vi "STED Control V10.vi"() -> ()   [LabVIEW 2014]
uses:
  Type Defs/Image Acquisition Parameters.ctl
  Laser Controls.ctl
  Detectors.ctl
  Type Defs/P541.ctl
  Type Defs/M227.ctl
  Type Defs/P612.ctl
  Type Defs/M686.ctl
  Type Defs/P841.ctl
  Type Defs/ASI.ctl
  Type Defs/N664_V2.ctl
  Type Defs/STED Graph Controls.ctl
  Type Defs/Display Controls.ctl
  FPGA-7842R-Reference.ctl
  Manual Controls V2.ctl
  Scan Parameters.ctl
  <vilib>/Utility/miscctls.llb/LVPositionTypeDef.ctl
  Controls/StageStates.ctl
  Focus Lock/Controls/Standard Action for Focus Lock.ctl
  <vilib>/Utility/miscctls.llb/LVRectTypeDef.ctl
  <vilib>/event_ctls.llb/lveventtype.ctl
  <vilib>/Utility/file.llb/Read From Spreadsheet File (DBL).vi
  <vilib>/Utility/file.llb/Write To Spreadsheet File (DBL).vi
panel:
  in  "Follow Cursor":bool
  in  "Laser Controls 2":T1={"Laser On Time (Ticks)"=16, "Laser Delay (Ticks)"=3}
  out "Channel 6":sgl[][](graph)
  out "Channel 5":sgl[][](graph)
  out "Channel 4":sgl[][](graph)
  out "Channel 3":sgl[][](graph)
  out "Channel 2":sgl[][](graph)
  out "Channel 1":sgl[][](graph)
  in  "Display Controls":T2
  in  "Graph Tools":T3={"Zoom Out"=FALSE, "Zoom In"=FALSE, "Reset Zoom"=FALSE, "Pan Tool"=FALSE, "Show Cursor"=FALSE, "Load File"=FALSE, "Fit Tool"=FALSE, "Smooth Tool"=FALSE, "Merge Tool"=FALSE, "Auto Scale"=FALSE, "Apply Color"=FALSE, "Color Map"=enum."Fire"}
  in  "Shutters":T4
  in  "Upper Objective Z - N664":T5={"Up N664"=FALSE, "Down N664"=FALSE, "Step Size (um)"=0.001, "Position (mm)"=0.0, "Home"=FALSE, "Save"=FALSE} {"Step Size (um)" min=0.001}
  in  "Cavity Translation Z - ASI":T6={"Up ASI"=FALSE, "Down ASI"=FALSE, "Step Size (um)"=0.001, "Z (um)"=0.001, "F (um)"=0.001, "Velocity"=0.001} caption="ASI" {"Velocity" min=0.001; "F (um)" min=0.001; "Z (um)" min=-1500.0 max=1500.0; "Step Size (um)" min=0.001}
  in  "Phase Comp Mirror - P841":T7={"Position (µm)"=0.0, "Step Size (µm)"=1.0, "Up P841"=FALSE, "Down P841"=FALSE}
  in  "Sample Stage XY - M686":T8={"Home Button"=FALSE, "Up Button"=FALSE, "Left Button"=FALSE, "Down Button"=FALSE, "Right Button"=FALSE, "X"=0.0, "Y"=0.0, "Step Size (um)"=1.0} {"Y" format="%#_8g"; "X" format="%#_8g"}
  in  "Bottom Objective XY - P612":T9
  in  "Abort AllStage":bool
  in  "Stages":T10={"M227"=TRUE, "N664"=TRUE, "P612"=TRUE, "M686"=TRUE, "P841"=TRUE, "ASI"=FALSE}
  in  "Sample Z Coarse - M227":T11
  in  "Tab Control":T12(tab)
  in  "SLM":bool
  in  "DM":bool
  in  "Timing":bool
  in  "Camera":bool
  in  "Focus Lock":bool
  in  "Sample Z - P541":T13={"Step Up"=FALSE, "Step Down"=FALSE, "Z Position"=0.0, "Step Size (um)"=1.0, "Home"=FALSE, "Save"=FALSE}
  in  "Detectors":T14={"PMT"=TRUE, "Far Red (685/40 nm)"=FALSE, "Orange (624/40 nm)"=FALSE, "Green (525/50 nm)"=FALSE, "Sum All"=FALSE}
  in  "Laser Controls":T15 {"STED Power (V)" scale=0.0..10.0}
  in  "Save File Path":path=path "C:/isoSTED_Data/Temp/Test_0000.dbl"
  in  "Capture":bool
  in  "Image Acquisition Parameters":T16={"Scan Type"=enum."Beam Scanning", "Scan Mode"=enum."XY", "Fast Axis Frequency (Hz)"=15780.0, "Image Format"=256, "Line Accumulations"=100, "Frames Per Capture"=1, "Frames Accumulations"=1, "Image Dimension (um)"=[15.0, 15.0], "Number of Z Steps"=1, "Z Steps Size (um)"=1.0, "Pixel Size (nm)"=[58.59375, 58.59375]} {"Z Steps Size (um)" min=0.0; "Number of Z Steps" min=1; "Frames Accumulations" min=1; "Frames Per Capture" min=1; "Line Accumulations" min=1; "Image Format" items=["64 x 64"=64, "128 x 128"=128, "256 x 256"=256, "512 x 512"=512, "1024 x 1024"=1024, "2048 x 2048"=2048]}
  in  "Live":bool
  in  "Exit":bool
  # "XY"
  # "Z"
  # "Length"
  # "Height"
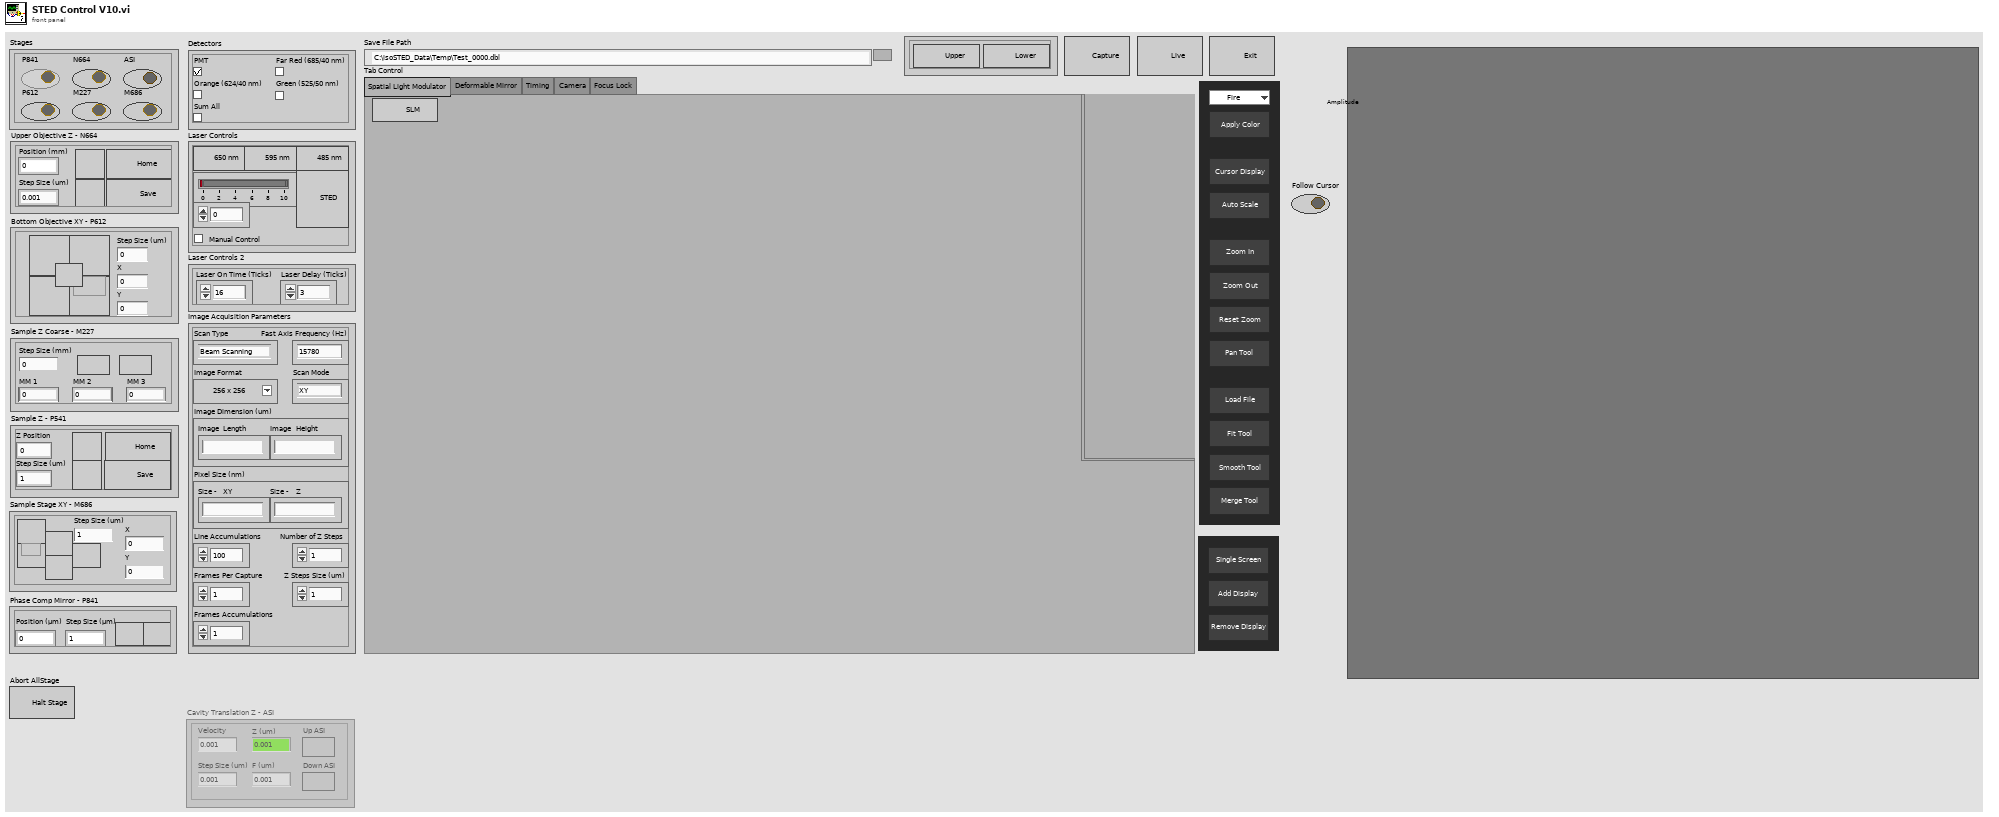
[diagram p1: front panel]
types:
  T1 = cluster{"Laser On Time (Ticks)":i8, "Laser Delay (Ticks)":i8}
  T2 = typedef "Display Controls.ctl" = cluster{"Remove Display":bool, "Add Display":bool, "Single Screen":bool}
  T3 = typedef "STED Graph Controls.ctl" = cluster{"Zoom Out":bool, "Zoom In":bool, "Reset Zoom":bool, "Pan Tool":bool, "Show Cursor":bool, "Load File":bool, "Fit Tool":bool, "Smooth Tool":bool, "Merge Tool":bool, "Auto Scale":bool, "Apply Color":bool, "Color Map":enum16{"System", "Fire", "Gray", "Red", "Green", "Blue", "Cyan", "Magenta", "Yellow", "Red-White", "Green-White", "Blue-White", "Glow"}}
  T4 = cluster{"Upper Shutter":bool, "Lower Shutter":bool}
  T5 = typedef "N664_V2.ctl" = cluster{"Up N664":bool, "Down N664":bool, "Step Size (um)":dbl, "Position (mm)":dbl, "Home":bool, "Save":bool}
  T6 = typedef "ASI.ctl" = cluster{"Up ASI":bool, "Down ASI":bool, "Step Size (um)":dbl, "Z (um)":dbl, "F (um)":dbl, "Velocity":dbl}
  T7 = typedef "P841.ctl" = cluster{"Position (µm)":dbl, "Step Size (µm)":dbl, "Up P841":bool, "Down P841":bool}
  T8 = typedef "M686.ctl" = cluster{"Home Button":bool, "Up Button":bool, "Left Button":bool, "Down Button":bool, "Right Button":bool, "X":dbl, "Y":dbl, "Step Size (um)":dbl}
  T9 = typedef "P612.ctl" = cluster{"Home Button":bool, "Up Button":bool, "Left Button":bool, "Down Button":bool, "Right Button":bool, "Step Size (um)":dbl, "X":dbl, "Y":dbl}
  T10 = cluster{"M227":bool, "N664":bool, "P612":bool, "M686":bool, "P841":bool, "ASI":bool}
  T11 = typedef "M227.ctl" = cluster{"Up M227":bool, "Down M227":bool, "Step Size (mm)":dbl, "MM 1":dbl, "MM 2":dbl, "MM 3":dbl}
  T12 = enum32{"Spatial Light Modulator", "Deformable Mirror", "Timing", "Camera", "Focus Lock"}
  T13 = typedef "P541.ctl" = cluster{"Step Up":bool, "Step Down":bool, "Z Position":dbl, "Step Size (um)":dbl, "Home":bool, "Save":bool}
  T14 = typedef "Detectors.ctl" = cluster{"PMT":bool, "Far Red (685/40 nm)":bool, "Orange (624/40 nm)":bool, "Green (525/50 nm)":bool, "Sum All":bool}
  T15 = typedef "Laser Controls.ctl" = cluster{"STED Power (V)":dbl, "STED":bool, "650 nm":bool, "590 nm":bool, "485 nm":bool, "Manual Control":bool}
  T16 = typedef "Image Acquisition Parameters.ctl" = cluster{"Scan Type":enum16{"Sample Scanning", "Beam Scanning"}, "Scan Mode":enum16{"XY", "XZ", "YZ", "XYZ"}, "Fast Axis Frequency (Hz)":dbl, "Image Format":u16, "Line Accumulations":u16, "Frames Per Capture":u16, "Frames Accumulations":u16, "Image Dimension (um)":dbl[], "Number of Z Steps":u8, "Z Steps Size (um)":dbl, "Pixel Size (nm)":dbl[]}
  T17 = typedef "Scan Parameters.ctl" = cluster{"Fast_Ax_Amp_V":dbl, "Fast_Ax_Off_V":dbl, "Slow_Ax_Amp_V":dbl, "Slow_Ax_Off_V ":dbl, "Slow_Ax_Max_V_VperS":dbl, "Slow_Ax1_Del25ns":i32, "Slow_Ax2_Del25ns":i32, "Stage_X_Off_V":dbl, "Stage_Y_Off_V":dbl, "Stage_Z_Off_V":dbl, "Galvo1_Off_V":dbl, "Galvo2_Off_V":dbl, "Last_Scan_Mode":enum16{"XY", "XZ", "YZ", "XYZ"}, "Current_Scan_Mode":enum16{"XY", "XZ", "YZ", "XYZ"}, "Fly_Back_Lines":u16, "Linear_Ramp_End":u32, "Z_Step_I16":i16, "Z_Start_I16":i16, "Laser_States _U32":u32, "590_Voltage_I16":i16, "775_AOM_Volt_I16":i16, "Blanking OFF":bool, "Unused_Axis_I16":i16}
  T18 = typedef "Manual Controls V2.ctl" = cluster{"Galvo 1 Position (I16)":i16, "Galvo 2 Position (I16)":i16, "X Axis Voltage (I16)":i16, "Y Axis Voltage (I16)":i16, "Z Axis Voltage (I16)":i16, "Res Mirror Amp (I16)":i16, "Res Mirror Mute":bool, "Upper Shutter":bool, "Lower Shutter":bool}
  T19 = typedef "FPGA-7842R-Reference.ctl" = enum16{"Stage Control", "Laser Control", "Unused Axis I16", "Exit", "Set Res Mirror", "Set Galvo", "Current Frame for Capture", "Default", "Close FPGA", "Stop Waveforms", "Start Waveforms", "Shutter Control", "Initialize"}
  T20 = enum8{"Enabled", "Disabled", "Disabled and Grayed Out"}
  T21 = typedef "StageStates.ctl" = enum16{"POSITION", "MVR", "MOVE", "HALT", "ONTARGET", "ERROR", "EXIT", "HOME", "ZEROPOS", "NANOPOS", "QUIT", "ANALOG"}
  T22 = typedef "Standard Action for Focus Lock.ctl" = enum16{"Read", "Write"}
  T23 = typedef "LVRectTypeDef.ctl" = cluster{"Left":i16, "Top":i16, "Right":i16, "Bottom":i16}
  T24 = enum32{"Invalid", "Standard", "Closed", "Hidden", "Minimized", "Maximized"}
  T25 = typedef "lveventtype.ctl" = enum32{"Null", "Timeout", "Annotation Menu Selection", "Annotation Menu Selection?", "App Instance Close", "App Instance Close?", "Autoscale Range Change", "Bookmark Info Change", "Cell Edit", "Cell Edit?", "Cursor Grab", "Cursor Grab?", "Cursor Menu Selection", "Cursor Menu Selection?", "Cursor Move", "Cursor Release", "Data Change", "Direction Change", "Display State Change", "Drag Ended", "Drag Enter", "Drag Leave", "Drag Over", "Drag Source Update", "Drag Starting", "Drag Starting?", "Drop", "Exec State Change", "Key Down", "Key Down?", "Key Repeat", "Key Repeat?", "Key Up", "Listbox Double Click", "Menu Activation?", "Menu Selection (App)", "Menu Selection? (App)", "Menu Selection (User)", "Mouse Down", "Mouse Down?", "Mouse Enter", "Mouse Leave", "Mouse Move", "Mouse Up", "Mouse Wheel", "NI Security User Change (App)", "Pane Size", "Panel Close", "Panel Close?", "Panel Resize", "Plot Attribute Change", "Scale Range Change", "Shortcut Menu Activation?", "Shortcut Menu Selection (App)", "Shortcut Menu Selection? (App)", "Shortcut Menu Selection (User)", "Tree Double Click", "Tree Drag", "Tree Drag?", "Tree Drop", "Tree Drop?", "Tree Item Close", "Tree Item Close?", "Tree Item Open", "Tree Item Open?", "User Event", "Value Change"}
  T26 = typedef "LVPositionTypeDef.ctl" = cluster{"Left":i32, "Top":i32}
  T27 = cluster{"Upper Shutter":bool, "Upper Shutter":bool}
  T28 = cluster{bool, bool, dbl, "Numeric":dbl, "Numeric":dbl, "Numeric":dbl}
  T29 = cluster{"Down_N664":bool, "Down_N664":bool, "Step Size (um)":dbl, "Numeric":dbl, bool, bool}
  T30 = cluster{bool, bool, bool, bool, bool, dbl, "Numeric":dbl, "Numeric":dbl}
  T31 = cluster{bool, bool, bool, bool, bool, "Numeric":dbl, "Numeric":dbl, dbl}
  T32 = cluster{"Scan Type":bool, "Scan Mode":bool, "Fast Axis Frequency (Hz)":bool, "Image Format":bool, "Line Accumulations":bool, "Frames Per Capture":bool, "Frames Accumulations":bool, "Image Dimension (um)":bool[], "Number of Z Steps":bool, "Z Steps Size (um)":bool, "Pixel Size (nm)":bool[]}
  T33 = cluster{"EXIT":bool, "Lock Current":bool, "Correct":bool, "Drift":bool, "Move":bool}
  T34 = typedef "LVAllMonitorsDisplayTypeDef.ctl" = cluster{"Bounds":cluster{"Left":i16, "Top":i16, "Right":i16, "Bottom":i16}, "Depth":i16}[]
  T35 = cluster{"Bounds":cluster{"Left":i16, "Top":i16, "Right":i16, "Bottom":i16}, "Depth":i16}
  T36 = enum16{"System", "Fire", "Gray", "Red", "Green", "Blue", "Cyan", "Magenta", "Yellow", "Red-White", "Green-White", "Blue-White", "Glow"}
  T37 = typedef "LVPointDoubleTypeDef.ctl" = cluster{"Cursor X":dbl, "Cursor Y":dbl}
  T38 = typedef "LVRangeTypeDef.ctl" = cluster{"Minimum":dbl, "Maximum":dbl, "Increment":dbl, "Minor Increment":dbl, "Start":dbl}
  T39 = typedef "IMAQ Image.ctl" = refnum<image>
  T40 = typedef "Waveform Data.ctl" = cluster{"Waveform Scan Parameters":cluster{"Scanning Mode":u8, "Fast Axis WF Length (Elements)":i32, "Fast Axis Sample Period (Ticks)":u32, "Slow Axis 1 WF Length (Elements)":i32, "Slow Axis 1 Sample Period (Ticks)":u32, "Slow Axis 1 Delay (25 ns) Steps":i32, "Slow Axis 2 WFLength (Elements)":i32, "Slow Axis 2 Sample Period (Ticks)":u32, "Slow Axis 2 Delay (25 ns) Steps":i32}, "Fast Axis Waveform":dbl[], "Slow Axis 1 Waveform":dbl[], "Slow Axis 2 Waveform":dbl[]}
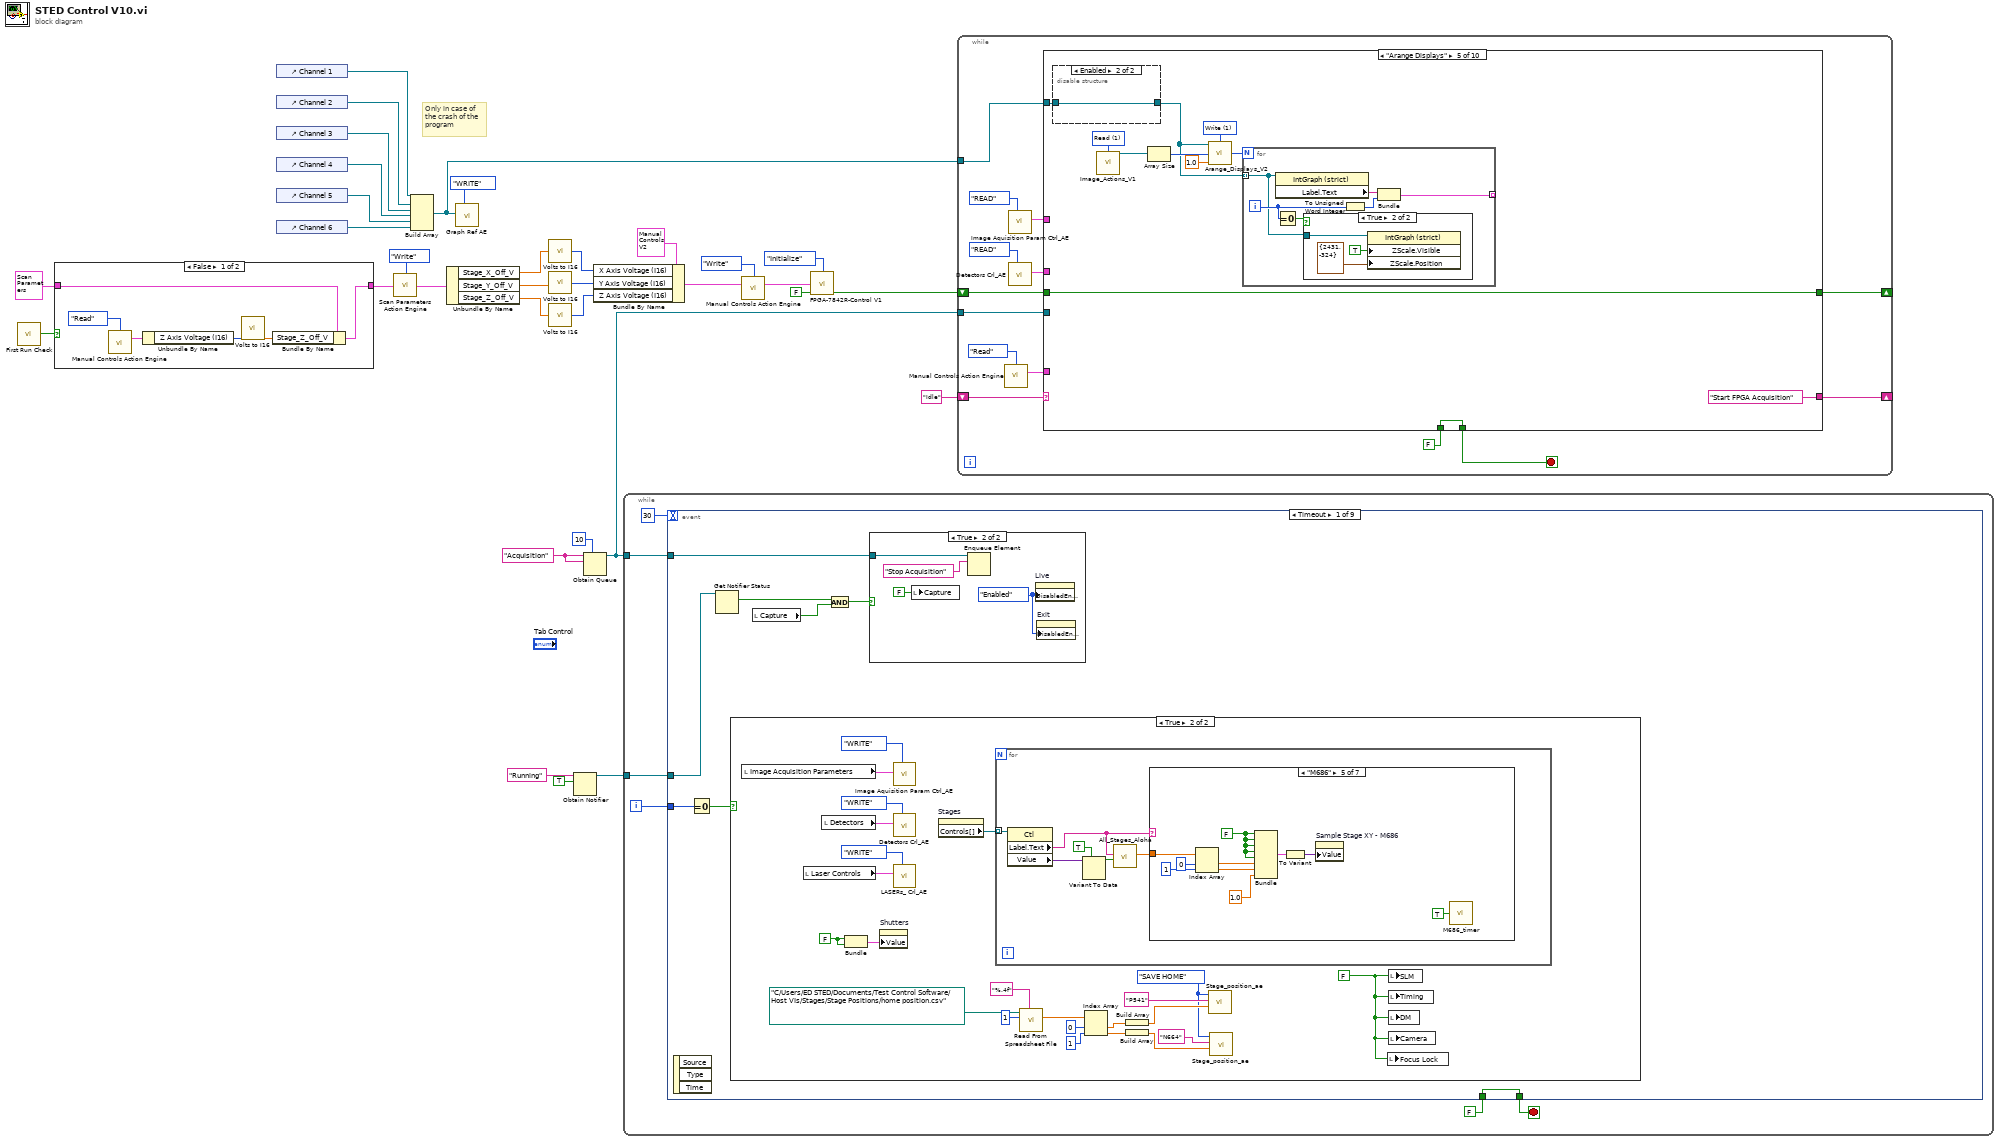
[diagram p0: block diagram]
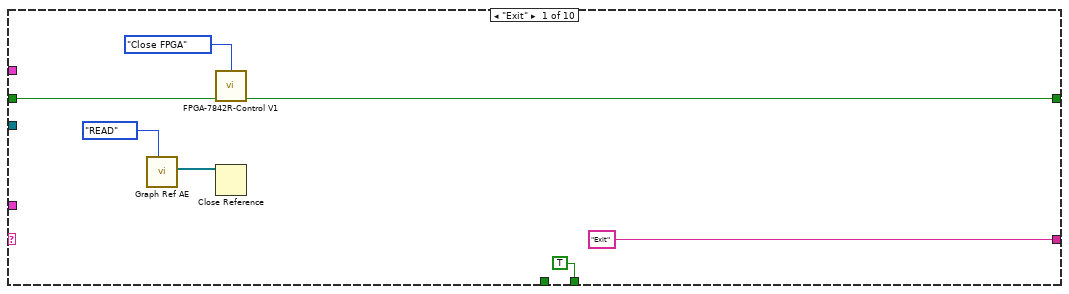
[diagram p3: hidden frame]
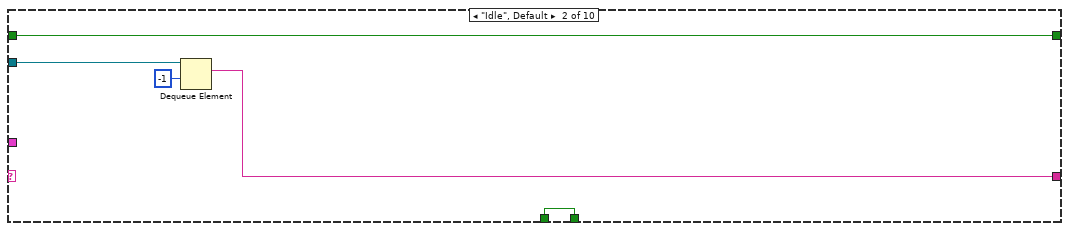
[diagram p4: hidden frame]
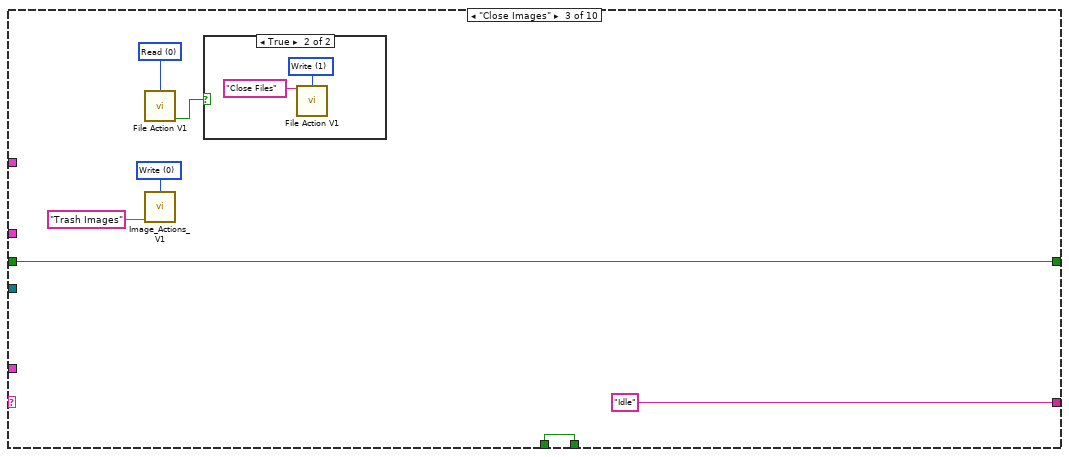
[diagram p5: hidden frame]
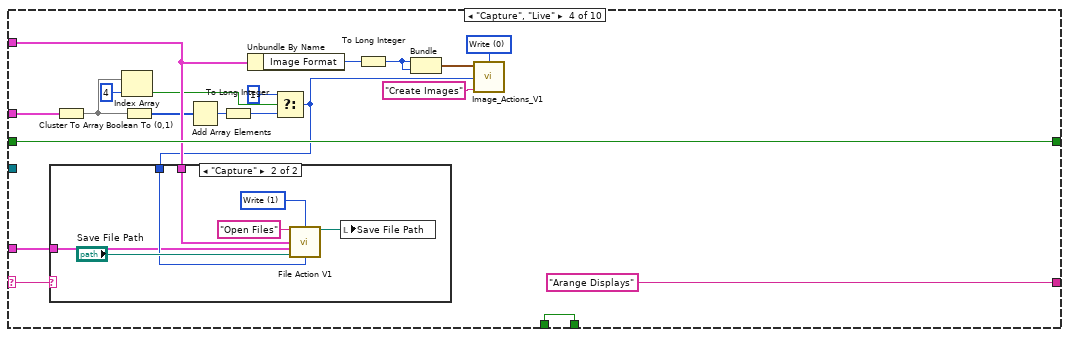
[diagram p7: hidden frame]
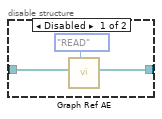
[diagram p9: hidden frame]
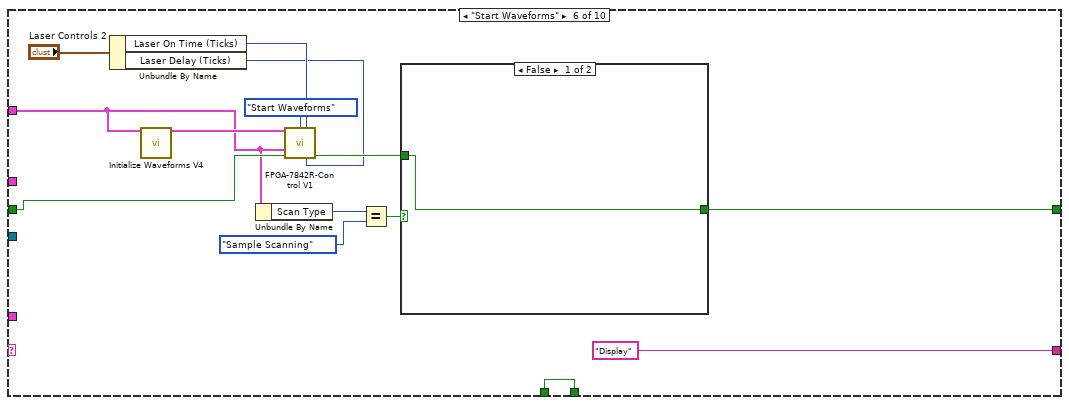
[diagram p11: hidden frame]
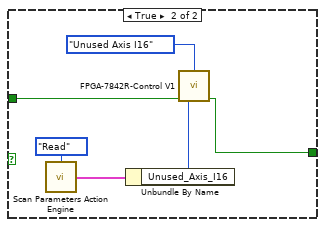
[diagram p12: hidden frame]
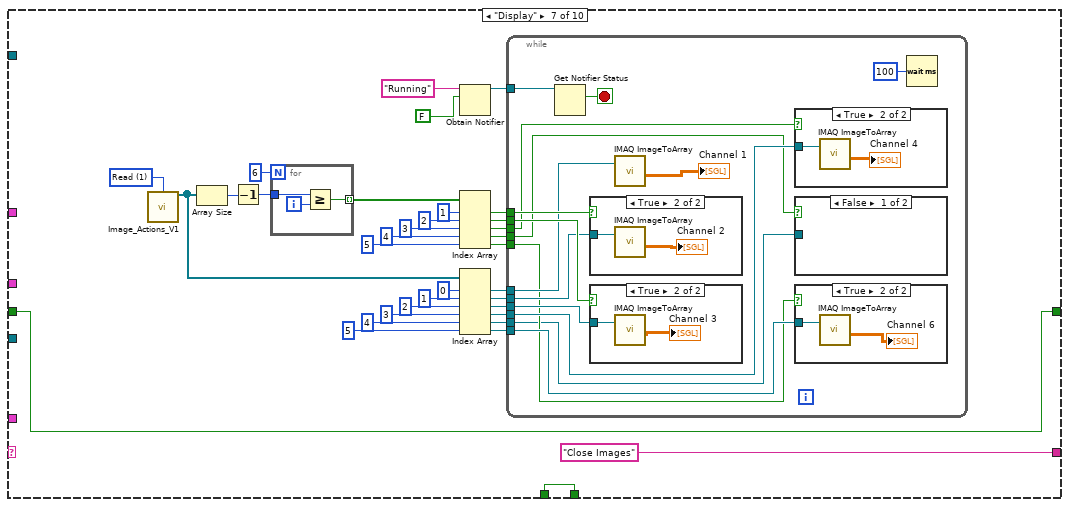
[diagram p13: hidden frame]
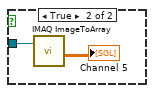
[diagram p15: hidden frame]
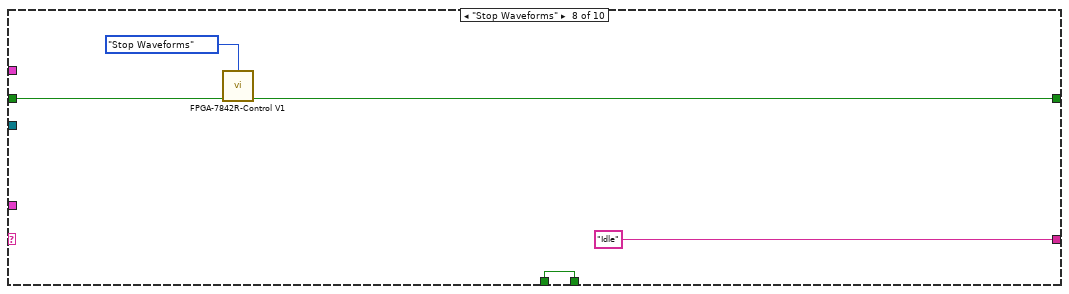
[diagram p19: hidden frame]
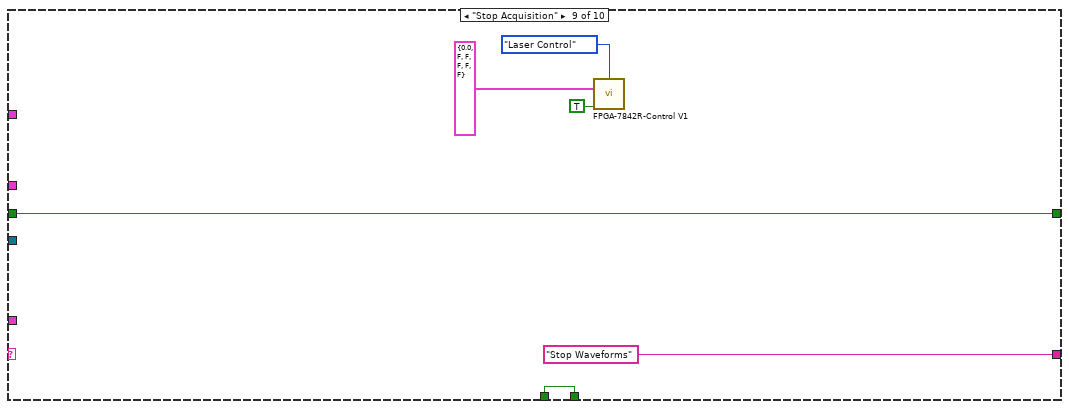
[diagram p20: hidden frame]
diagram:
  w16 = "Acquisition" ("name (unnamed)")
  # "Only in case of \nthe crash of the\nprogram"
  n1 = call "First Run Check.vi"() -> ("First Run?"=w10:bool)  [unwired: 15 in]
  n2 = case shown="False" w10 {
    tunnel: T17 {"Fast_Ax_Amp_V"=0.0, "Fast_Ax_Off_V"=0.0, "Slow_Ax_Amp_V"=0.0, "Slow_Ax_Off_V "=0.0, "Slow_Ax_Max_V_VperS"=0.0, "Slow_Ax1_Del25ns"=0, "Slow_Ax2_Del25ns"=0, "Stage_X_Off_V"=5.0, "Stage_Y_Off_V"=5.0, "Stage_Z_Off_V"=5.0, "Galvo1_Off_V"=0.0, "Galvo2_Off_V"=0.0, "Last_Scan_Mode"=enum."XY", "Current_Scan_Mode"=enum."XY", "Fly_Back_Lines"=0, "Linear_Ramp_End"=0, "Z_Step_I16"=0, "Z_Start_I16"=0, "Laser_States _U32"=0, "590_Voltage_I16"=0, "775_AOM_Volt_I16"=0, "Blanking OFF"=FALSE, "Unused_Axis_I16"=16384} ("Scan Parameters IN") -> [w39 w40]
    tunnel: [w34 w40] -> w8
    frame False {
      n3 = call "Manual Controls Action Engine.vi"("Action"=enum16{"Read", "Write"}."Read") -> ("Manual Controls Out"=w37:T18)  [unwired: 14 in]
      n4 = Unbundle By Name(w37) -> ("Z Axis Voltage (I16)"=w38:i16)
      n5 = call "Volts to I16.vi"("Volatge (I16)"=w38) -> ("Voltage (V)"=w35:dbl)  [unwired: 13 in, 1 out]
      n6 = Bundle By Name(cluster=w39, "Stage_Z_Off_V"=w35) -> (w34:T17)
    }
    frame True {
    }
  }
  n7 = control-ref of="Channel 1"() -> (w5:refnum<vi>)
  n8 = control-ref of="Channel 2"() -> (w6:refnum<vi>)
  n9 = control-ref of="Channel 3"() -> (w7:refnum<vi>)
  n10 = control-ref of="Channel 4"() -> (w2:refnum<vi>)
  n11 = control-ref of="Channel 5"() -> (w4:refnum<vi>)
  n12 = control-ref of="Channel 6"() -> (w3:refnum<vi>)
  n13 = call "Scan Parameters Action Engine.vi"("Action"=enum16{"Read", "Write"}."Write", "Scan Parameters IN"=w8) -> ("Scan Parameters OUT"=w26:T17)  [unwired: 13 in]
  n14 = Build Array(w5, w6, w7, w2, w4, w3) -> (w1:refnum<vi>[])
  n15 = Unbundle By Name(w26) -> ("Stage_X_Off_V"=w22:dbl, "Stage_Y_Off_V"=w21:dbl, "Stage_Z_Off_V"=w20:dbl)
  n16 = call "Graph Ref AE.vi"("Action"=enum16{"READ", "WRITE"}."WRITE", "Graph Ref In"=w1) -> ()  [unwired: 9 in, 1 out]
  n17 = call "Volts to I16.vi"("Voltage (V)"=w22) -> ("I16"=w23:i16)  [unwired: 13 in, 1 out]
  n18 = call "Volts to I16.vi"("Voltage (V)"=w21) -> ("I16"=w24:i16)  [unwired: 13 in, 1 out]
  n19 = call "Volts to I16.vi"("Voltage (V)"=w20) -> ("I16"=w25:i16)  [unwired: 13 in, 1 out]
  n20 = Obtain Notifier(name (unnamed)="Running", notification data type=TRUE) -> (notifier out=w12:refnum<notifier>)  [unwired: 2 in, 2 out]
  n21 = Obtain Queue(max queue size (-1, unlimited)=10, name (unnamed)=w16, element data type=w16) -> (queue out=w18:refnum<queue>)  [unwired: 2 in, 2 out]
  n22 = Bundle By Name(cluster=T18 {"Galvo 1 Position (I16)"=-280, "Galvo 2 Position (I16)"=0, "X Axis Voltage (I16)"=16384, "Y Axis Voltage (I16)"=16384, "Z Axis Voltage (I16)"=16384, "Res Mirror Amp (I16)"=0, "Res Mirror Mute"=FALSE, "Upper Shutter"=FALSE, "Lower Shutter"=FALSE} ("Manual Controls"), "X Axis Voltage (I16)"=w23, "Y Axis Voltage (I16)"=w24, "Z Axis Voltage (I16)"=w25) -> (w27:T18)
  n23 = while {
    tunnel: w18 -> [w44]
    tunnel: w12 -> [w41]
    i -> [w42]
    stop <- w46 stop-if-true
    n24 = event shown="[0] Timeout" {
      selector: _ -> [_ _ _ _ _ _ _ _ _]
      dyn-events: _ -> [_ _ _ _ _ _ _ _ _]
      timeout: 30 -> [_ _ _ _ _ _ _ _ _]
      tunnel: [w54 w189 w202 w367 _ w714 w795 w999 w1052] -> w46
      tunnel: FALSE -> [w54 w189 w202 w367 _ w714 w795 w999 _]
      tunnel: w44 -> [w51 w188 _ _ _ _ _ _ w1051]
      tunnel: w42 -> [w49 _ _ _ _ _ _ _ _]
      tunnel: w41 -> [w47 w181 _ _ _ _ _ _ w1045]
      event Timeout {
        n25 = event-data() -> ()  [unwired: 1 in, 3 out]
        n26 = Equal To 0?(x=w49) -> (x = 0?=w48:bool)
        n27 = Get Notifier Status(notifier=w47) -> (current notification=w53:bool)  [unwired: 1 in, 4 out]
        n28 = case shown="True" w48 {
          frame False {
            w61 = enum16{"WRITE", "READ", "HOME", "SAVE HOME"}."READ" ("Enum")
            n29 = call "Image Aquisition Param Ctrl_AE.vi"("Action"=enum16{"READ", "WRITE"}."READ") -> ("Image Acquisition Parameters Out"=w89:T16)  [unwired: 10 in]
            n30 = call "Detectors Crl_AE.vi"("Action"=enum16{"READ", "WRITE"}."READ") -> ("Detectors Parameters Out"=w90:T14)  [unwired: 10 in]
            n31 = call "LASERs_ Crl_AE.vi"("Action"=enum16{"READ", "WRITE"}."READ") -> ("Detectors Parameters Out"=w91:T15)  [unwired: 10 in]
            n32 = local write "Image Acquisition Parameters"(w89) -> ()
            n33 = local write "Detectors"(w90) -> ()
            n34 = local write "Laser Controls"(w91) -> ()
            n35 = call "Stage_position_ae.vi"("StageID"="M686", "Enum"=w61) -> ("Position Out"=w59:dbl[])  [unwired: 8 in, 1 out]
            n36 = call "Stage_position_ae.vi"("StageID"="M227", "Enum"=w61) -> ("Position Out"=w67:dbl[])  [unwired: 8 in, 1 out]
            n37 = call "Stage_position_ae.vi"("StageID"="P612", "Enum"=w61) -> ("Position Out"=w84:dbl[])  [unwired: 8 in, 1 out]
            n38 = call "Stage_position_ae.vi"("StageID"="P841", "Enum"=w61) -> ("Position Out"=w77:dbl[])  [unwired: 8 in, 1 out]
            n39 = call "Stage_position_ae.vi"("StageID"="N664", "Enum"=w61) -> ("Position Out"=w71:dbl[])  [unwired: 8 in, 1 out]
            n40 = Index Array(array=w71, index=0) -> (element=w70:dbl)
            n41 = Index Array(array=w77, index=0) -> (element=w74:dbl)
            n42 = Index Array(array=w84, index #1=0 ("index"), index #2=1 ("index"), index #3=2 ("index")) -> (element #1=w83:dbl, element #2=w80:dbl, element #3=w78:dbl)
            n43 = Index Array(array=w59, index #1=0 ("index"), index #2=1 ("index")) -> (element #1=w56:dbl, element #2=w55:dbl)
            n44 = Index Array(array=w67, index #1=0 ("index"), index #2=1 ("index"), index #3=2 ("index")) -> (element #1=w64:dbl, element #2=w63:dbl, element #3=w62:dbl)
            n45 = property on="Position (µm)" class="DigNum (strict)"("Value"=w74) -> ()  [unwired: 2 in, 2 out]
            n46 = property on="Position (mm)" class="DigNum (strict)"("Value"=w70) -> ()  [unwired: 2 in, 2 out]
            n47 = property on="X" class="DigNum (strict)"("Value"=w83) -> ()  [unwired: 2 in, 2 out]
            n48 = property on="Y" class="DigNum (strict)"("Value"=w80) -> ()  [unwired: 2 in, 2 out]
            n49 = property on="X" class="DigNum (strict)"("Value"=w56) -> ()  [unwired: 2 in, 2 out]
            n50 = property on="MM 1" class="DigNum (strict)"("Value"=w64) -> ()  [unwired: 2 in, 2 out]
            n51 = property on="MM 2" class="DigNum (strict)"("Value"=w63) -> ()  [unwired: 2 in, 2 out]
            n52 = property on="Z Position" class="DigNum (strict)"("Value"=w78) -> ()  [unwired: 2 in, 2 out]
            n53 = property on="Y" class="DigNum (strict)"("Value"=w55) -> ()  [unwired: 2 in, 2 out]
            n54 = property on="MM 3" class="DigNum (strict)"("Value"=w62) -> ()  [unwired: 2 in, 2 out]
          }
          frame True {
            w92 = FALSE ("SLM")
            w94 = enum16{"WRITE", "READ", "HOME", "SAVE HOME"}."SAVE HOME" ("Enum")
            w106 = FALSE ("Upper Shutter")
            n55 = local read "Image Acquisition Parameters"() -> (w113:T16)
            n56 = local read "Laser Controls"() -> (w111:T15)
            n57 = local read "Detectors"() -> (w110:T14)
            n58 = Bundle("Upper Shutter"=w106, "Upper Shutter"=w106) -> (w107:T27)  [unwired: 1 in]
            n59 = property on="Shutters" class="Clust (strict)"("Value"=w107) -> ()  [unwired: 2 in, 2 out]
            n60 = call "Image Aquisition Param Ctrl_AE.vi"("Action"=enum16{"READ", "WRITE"}."WRITE", "Image Acquisition Parameters In"=w113) -> ()  [unwired: 9 in, 1 out]
            n61 = call "Detectors Crl_AE.vi"("Action"=enum16{"READ", "WRITE"}."WRITE", "Detectors Parameters In"=w110) -> ()  [unwired: 9 in, 1 out]
            n62 = call "LASERs_ Crl_AE.vi"("Action"=enum16{"READ", "WRITE"}."WRITE", "Detectors Parameters In"=w111) -> ()  [unwired: 9 in, 1 out]
            n63 = property on="Stages" class="Clust (strict)"() -> ("Controls[]"=w108:refnum<vi>[])  [unwired: 2 in, 2 out]
            n64 = for {
              tunnel: w108 -> [w118] mode=indexing
              n65 = property class="Ctl"(reference=w118) -> ("Label.Text"=w116:string, "Value"=w120:variant)  [unwired: 1 in, 2 out]
              n66 = Variant To Data(type=TRUE, Variant=w120) -> (data=w117:bool)  [unwired: 1 in, 1 out]
              n67 = call "All_Stages_Aloha.vi"("Aloha"=w117, "Stage ID"=w116) -> ("Position Out"=w115:dbl[])  [unwired: 9 in]
              n68 = case shown="\"M686\"" w116 {
                tunnel: w115 -> [_ w127 w135 w142 w151 w162 w172]
                frame "0", Default {
                }
                frame "M227" {
                  w131 = FALSE
                  n69 = Index Array(array=w127, index #1=0 ("index"), index #2=1 ("index"), index #3=2 ("index")) -> (element #1=w123:dbl, element #2=w122:dbl, element #3=w121:dbl)
                  n70 = Bundle(w131, w131, 0.0, "Numeric"=w123, "Numeric"=w122, "Numeric"=w121) -> (w129:T28)  [unwired: 1 in]
                  n71 = To Variant(anything=w129) -> (Variant=w128:variant)
                  n72 = property on="Sample Z Coarse - M227" class="Clust"("Value"=w128) -> ()  [unwired: 2 in, 2 out]
                }
                frame "N664" {
                  w132 = FALSE
                  w138 = FALSE ("Down_N664")
                  n73 = Index Array(array=w135, index=0) -> (element=w136:dbl)
                  n74 = Bundle("Down_N664"=w138, "Down_N664"=w138, "Step Size (um)"=1.0, "Numeric"=w136, w132, w132) -> (w134:T29)  [unwired: 1 in]
                  n75 = To Variant(anything=w134) -> (Variant=w133:variant)
                  n76 = property on="Upper Objective Z - N664" class="Clust"("Value"=w133) -> ()  [unwired: 2 in, 2 out]
                }
                frame "P612" {
                  w150 = FALSE
                  n77 = Index Array(array=w142, index #1=0, index #2=1, index #3=2 ("index")) -> (element #1=w147:dbl, element #2=w145:dbl, element #3=w140:dbl)
                  n78 = Bundle(w150, w150, w150, w150, w150, 1.0, "Numeric"=w147, "Numeric"=w145) -> (w146:T30)  [unwired: 1 in]
                  n79 = To Variant(anything=w146) -> (Variant=w141:variant)
                  n80 = property on="Bottom Objective XY - P612" class="Clust"("Value"=w141) -> ()  [unwired: 2 in, 2 out]
                  n81 = property on="Z Position" class="DigNum (strict)"("Value"=w140) -> ()  [unwired: 2 in, 2 out]
                }
                frame "M686" {
                  w160 = FALSE
                  n82 = Index Array(array=w151, index #1=0, index #2=1) -> (element #1=w155:dbl, element #2=w154:dbl)
                  n83 = Bundle(w160, w160, w160, w160, w160, "Numeric"=w155, "Numeric"=w154, 1.0) -> (w158:T31)  [unwired: 1 in]
                  n84 = To Variant(anything=w158) -> (Variant=w156:variant)
                  n85 = property on="Sample Stage XY - M686" class="Clust"("Value"=w156) -> ()  [unwired: 2 in, 2 out]
                  n86 = call "M686_timer.vi"("Reset"=TRUE) -> ()  [unwired: 1 out]
                }
                frame "P841" {
                  n87 = Index Array(array=w162, index=0) -> (element=w161:dbl)
                  n88 = property on="Position (µm)" class="DigNum (strict)"("Value"=w161) -> ()  [unwired: 2 in, 2 out]
                }
                frame "ASI" {
                  w168 = FALSE
                  n89 = Add Array Elements(numeric array=w172) -> (sum=w174:dbl)
                  n90 = Index Array(array=w172, index #1=0 ("index"), index #2=1 ("index")) -> (element #1=w167:dbl, element #2=w166:dbl)
                  n91 = Divide(x=w174, y=2000.0) -> ()  [unwired: 1 out]
                  n92 = Bundle By Name(cluster=T6 {"Up ASI"=FALSE, "Down ASI"=FALSE, "Step Size (um)"=0.001, "Z (um)"=0.001, "F (um)"=0.001, "Velocity"=0.001} ("Cavity Translation Z - ASI"), "Up ASI"=w168, "Down ASI"=w168, "Step Size (um)"=1.0, "Z (um)"=w167, "F (um)"=w166, "Velocity"=0.1) -> (w164:T6)
                  n93 = To Variant(anything=w164) -> (Variant=w165:variant)
                  n94 = property on="Cavity Translation Z - ASI" class="Clust"("Value"=w165) -> ()  [unwired: 2 in, 2 out]
                }
              }
            }
            n95 = call-poly <vilib>:"Read From Spreadsheet File.vi"("format (%.3f)"="%.4f", "number of rows (all:-1)"=1, "file path (dialog if empty)"=path "C:/Users/ED STED/Documents/Test Control Software/Host VIs/Stages/Stage Positions/home position.csv") -> ("first row"=w103:dbl[])  [unwired: 4 in, 4 out]
            n96 = Index Array(array=w103, index #1=0 ("index"), index #2=1 ("index")) -> (element #1=w99:dbl, element #2=w100:dbl)
            n97 = Build Array(w99) -> (w98:dbl[])
            n98 = Build Array(w100) -> (w96:dbl[])
            n99 = call "Stage_position_ae.vi"("Position In"=w98, "StageID"="P541", "Enum"=w94) -> ()  [unwired: 7 in, 2 out]
            n100 = call "Stage_position_ae.vi"("Position In"=w96, "StageID"="N664", "Enum"=w94) -> ()  [unwired: 7 in, 2 out]
            n101 = local write "Focus Lock"(w92) -> ()
            n102 = local write "SLM"(w92) -> ()
            n103 = local write "Timing"(w92) -> ()
            n104 = local write "DM"(w92) -> ()
            n105 = local write "Camera"(w92) -> ()
          }
        }
        n106 = local read "Capture"() -> (w52:bool)
        n107 = And(x=w53, y=w52) -> (x .and. y?=w50:bool)
        n108 = case shown="True" w50 {
          tunnel: w51 -> [_ w179]
          frame False {
          }
          frame True {
            w177 = T20."Enabled" ("Disabled")
            n109 = local write "Capture"(FALSE ("Capture")) -> ()
            n110 = Enqueue Element(queue=w179, element="Stop Acquisition" ("f")) -> ()  [unwired: 2 in, 3 out]
            n111 = property on="Live" class="Bool (strict)"("DisabledEnum"=w177) -> ()  [unwired: 2 in, 2 out]
            n112 = property on="Exit" class="Bool"("DisabledEnum"=w177) -> ()  [unwired: 2 in, 2 out]
          }
        }
      }
      event "Live", "Capture": Value Change {
        n113 = event-data() -> ("CtlRef"=w187:refnum<vi>, "NewVal"=w182:bool)  [unwired: 1 in]
        n114 = Not(x=w182) -> (.not. x?=w185:bool)
        n115 = property class="Bool (strict)"(reference=w187) -> ("Label.Text"=w183:string)  [unwired: 1 in, 2 out]
        n116 = Send Notification(notification=w185, notifier=w181) -> ()  [unwired: 1 in, 2 out]
        n117 = case shown="\"Capture\"" w183 {
          tunnel: w182 -> [_ w191 w194]
          frame "False", Default {
          }
          frame "Live" {
            n118 = case shown="True" w191 {
              tunnel: [T20."Enabled" ("Disabled") T20."Disabled and Grayed Out" ("Disabled")] -> w190
              frame False {
              }
              frame True {
              }
            }
            n119 = property on="Capture" class="Bool (strict)"("DisabledEnum"=w190) -> ()  [unwired: 2 in, 2 out]
            n120 = property on="Exit" class="Bool"("DisabledEnum"=w190) -> ()  [unwired: 2 in, 2 out]
          }
          frame "Capture" {
            n121 = case shown="True" w194 {
              tunnel: [T20."Enabled" ("Disabled") T20."Disabled and Grayed Out" ("Disabled")] -> w195
              frame False {
              }
              frame True {
              }
            }
            n122 = property on="Live" class="Bool (strict)"("DisabledEnum"=w195) -> ()  [unwired: 2 in, 2 out]
            n123 = property on="Exit" class="Bool"("DisabledEnum"=w195) -> ()  [unwired: 2 in, 2 out]
          }
        }
        n124 = Select(t=w183, s=w182, f="Stop Acquisition") -> (s? t:f=w184:string)
        n125 = Enqueue Element(queue=w188, element=w184) -> ()  [unwired: 2 in, 3 out]
      }
      event "Shutters": Value Change {
        n126 = event-data() -> ("CtlRef"=w201:refnum<vi>, "NewVal"=w200:variant, "OldVal"=w199:variant)  [unwired: 1 in]
        n127 = property class="Clust"(reference=w201) -> ("Label.Text"=w198:string)  [unwired: 1 in, 2 out]
        n128 = case shown="\"Image Acquisition Parameters\"" w198 {
          tunnel: w200 -> [_ w217 _ _ _]
          tunnel: w199 -> [_ w215 _ _ _]
          frame Default {
          }
          frame "Image Acquisition Parameters" {
            n129 = Variant To Data(type="Image Acquisition Parameters", Variant=w217) -> (data=w214:T16)  [unwired: 1 in, 1 out]
            n130 = Variant To Data(type=w214, Variant=w215) -> (data=w213:T16)  [unwired: 1 in, 1 out]
            n131 = Not Equal?(x=w214, y=w213) -> (x != y?=w238:T32)
            n132 = Unbundle By Name(w238) -> ("Image Dimension (um)"=w223:bool[], "Image Format"=w221:bool, "Pixel Size (nm)"=w222:bool[], "Scan Mode"=w204:bool)
            n133 = Or Array Elements(Boolean array=w223) -> (logical OR=w227:bool)
            n134 = Or Array Elements(Boolean array=w222) -> (logical OR=w226:bool)
            n135 = Build Array(w227, w221, w226) -> (w225:bool[])
            n136 = Boolean Array To Number(Boolean array=w225) -> (number=w224:u32)
            n137 = case shown="1, 2" w224 {
              tunnel: w223 -> [_ w288 _]
              tunnel: w214 -> [w276 w281 w296]
              tunnel: [w276 w279 w294] -> w220
              tunnel: w222 -> [_ _ w293]
              tunnel: [w275 w278 w292] -> w219
              tunnel: [w274 w277 w291] -> w206
              frame 0, Default {
                n138 = Unbundle By Name(w276) -> ("Image Dimension (um)"=w275:dbl[], "Scan Mode"=w274:enum16{"XY", "XZ", "YZ", "XYZ"})
              }
              frame 1, 2 {
                # "Image Dimension or Format Change"
                n139 = Unbundle By Name(w281) -> ("Image Dimension (um)"=w287:dbl[], "Image Format"=w285:u16, "Scan Mode"=w277:enum16{"XY", "XZ", "YZ", "XYZ"})
                n140 = for {
                  tunnel: w288 -> [w290] mode=indexing
                  tunnel: w287 -> [w289] mode=indexing
                  tunnel: [w289] -> w286
                  stop <- w290 stop-if-true
                }
                n141 = To Double Precision Float(number=w285) -> (double precision float=w284:dbl)
                n142 = Build Array(w286, w286) -> (w278:dbl[])
                n143 = Divide(x=w278, y=w284) -> (x/y=w283:dbl[])
                n144 = Multiply(x=w283, y=1000.0) -> (x*y=w280:dbl[])
                n145 = Bundle By Name(cluster=w281, "Image Dimension (um)"=w278, "Pixel Size (nm)"=w280) -> (w279:T16)
              }
              frame 4 {
                # "Pixel Size Change"
                n146 = Unbundle By Name(w296) -> ("Pixel Size (nm)"=w302:dbl[], "Image Format"=w300:u16, "Scan Mode"=w291:enum16{"XY", "XZ", "YZ", "XYZ"})
                n147 = for {
                  tunnel: w293 -> [w304] mode=indexing
                  tunnel: w302 -> [w303] mode=indexing
                  tunnel: [w303] -> w301
                  stop <- w304 stop-if-true
                }
                n148 = Build Array(w301, w301) -> (w295:dbl[])
                n149 = To Double Precision Float(number=w300) -> (double precision float=w299:dbl)
                n150 = Multiply(x=w295, y=w299) -> (x*y=w298:dbl[])
                n151 = Multiply(x=w298, y=0.001) -> (x*y=w292:dbl[])
                n152 = Bundle By Name(cluster=w296, "Pixel Size (nm)"=w295, "Image Dimension (um)"=w292) -> (w294:T16)
              }
            }
            n153 = And(x=w204, y="Follow Cursor") -> (x .and. y?=w203:bool)
            n154 = case shown="True" w203 {
              tunnel: w206 -> [_ w248]
              frame False {
              }
              frame True {
                n155 = Not Equal?(x=w248, y=enum16{"XY", "XZ", "YZ", "XYZ"}."XZ") -> (x != y?=w246:bool)
                n156 = case shown="True" w246 {
                  frame False {
                    n157 = call "Y Slice.vi"() -> ("Y position"=w256:dbl)  [unwired: 1 in]
                    n158 = Build Array(0.0 ("element"), w256) -> (w254:dbl[])
                    n159 = call "AllStage_Limits_Array.vi"("Step(um)/Position(units)"=w254, "Axis"=bool[] [TRUE, TRUE, TRUE], "Stage ID"="M686", "MOVE/MVR"=enum16{"MOVE", "MVR"}."MVR") -> ("Positions"=w250:dbl[], "Boolean Array"=w251:bool[], "Stage ID"=w252:string)  [unwired: 4 in, 1 out]
                    n160 = call "AE_AllStages_Action V2.vi"("Velocity"=0.0, "Positions"=w250, "Axis"=w251, "Stage ID"=w252, "Action"=StageStates."MVR") -> ()  [unwired: 4 in, 3 out]
                  }
                  frame True {
                    n161 = call "Z Slice.vi"() -> ("Y position"=w270:dbl)  [unwired: 1 in]
                    n162 = call "Manual Controls Action Engine.vi"("Action"=enum16{"Read", "Write"}."Read") -> ("Manual Controls Out"=w265:T18)  [unwired: 14 in]
                    n163 = Multiply(x=w270, y=327.68) -> (x*y=w272:dbl)
                    n164 = Round To Nearest(number=w272) -> (nearest integer value=w271:dbl)
                    n165 = Unbundle By Name(w265) -> ("Z Axis Voltage (I16)"=w268:i16)
                    n166 = To Word Integer(number=w271) -> (16bit integer=w267:i16)
                    n167 = Add(x=w268, y=w267) -> (x+y=w266:i16)
                    n168 = Bundle By Name(cluster=w265, "Z Axis Voltage (I16)"=w266) -> (w264:T18)
                    n169 = call "Manual Controls Action Engine.vi"("Action"=enum16{"Read", "Write"}."Write", "Manual Controls In"=w264) -> ("Manual Controls Out"=w262:T18)  [unwired: 13 in]
                    n170 = call "FPGA-7842R-Control V1.vi"("Action"=FPGA-7842R-Reference."Stage Control", "Manual Controls"=w262, "Initialize"=TRUE) -> ()  [unwired: 11 in, 2 out]
                  }
                }
              }
            }
            n171 = Index Array(array=w219, index=0) -> (element=w243:dbl)
            n172 = Not Equal?(x=enum16{"XY", "XZ", "YZ", "XYZ"}."YZ" ("y"), y=w206) -> (x != y?=w228:bool)
            n173 = call "Res Mirror um to Volts.vi"("Image Size (um)"=w243) -> ("Voltage (V)"=w207:dbl)
            n174 = Select(t=15780.0, s=w228, f=200.0) -> (s? t:f=w231:dbl)
            n175 = In Range and Coerce(upper limit=5.0, x=w207, lower limit=0.0) -> (coerced(x)=w209:dbl)  [unwired: 1 out]
            n176 = call "Scan Parameters Action Engine.vi"("Action"=enum16{"Read", "Write"}."Read") -> ("Scan Parameters OUT"=w210:T17)  [unwired: 14 in]
            n177 = Bundle By Name(cluster=w210, "Fast_Ax_Amp_V"=w209) -> (w208:T17)
            n178 = Bundle By Name(cluster=w220, "Fast Axis Frequency (Hz)"=w231) -> (w230:T16)
            n179 = call "Volts to I16.vi"("Voltage (V)"=w209) -> ("I16"=w242:i16)  [unwired: 13 in, 1 out]
            n180 = call "Scan Parameters Action Engine.vi"("Action"=enum16{"Read", "Write"}."Write", "Scan Parameters IN"=w208) -> ()  [unwired: 13 in, 1 out]
            n181 = call "Manual Controls Action Engine.vi"("Action"=enum16{"Read", "Write"}."Read") -> ("Manual Controls Out"=w236:T18)  [unwired: 14 in]
            n182 = Bundle By Name(cluster=w236, "Res Mirror Amp (I16)"=w242, "Res Mirror Mute"=w228) -> (w234:T18)
            n183 = call "Image Aquisition Param Ctrl_AE.vi"("Action"=enum16{"READ", "WRITE"}."WRITE", "Image Acquisition Parameters In"=w230) -> ()  [unwired: 9 in, 1 out]
            n184 = call "FPGA-7842R-Control V1.vi"("Action"=FPGA-7842R-Reference."Set Res Mirror", "Manual Controls"=w234, "Initialize"=TRUE) -> ()  [unwired: 11 in, 2 out]
            n185 = call "Manual Controls Action Engine.vi"("Action"=enum16{"Read", "Write"}."Write", "Manual Controls In"=w234) -> ()  [unwired: 13 in, 1 out]
          }
          frame "Detectors" {
            n186 = call "Detectors Crl_AE.vi"("Action"=enum16{"READ", "WRITE"}."WRITE", "Detectors Parameters In"="Detectors") -> ()  [unwired: 9 in, 1 out]
          }
          frame "Laser Controls" {
            w319 = FALSE ("element")
            n187 = Unbundle By Name("Laser Controls") -> ("STED"=w325:bool, "650 nm"=w322:bool, "590 nm"=w323:bool, "485 nm"=w324:bool, "STED Power (V)"=w316:dbl, "Manual Control"=w308:bool)
            n188 = local read "Live"() -> (w311:bool)
            n189 = call "LASERs_ Crl_AE.vi"("Action"=enum16{"READ", "WRITE"}."WRITE", "Detectors Parameters In"="Laser Controls") -> ()  [unwired: 9 in, 1 out]
            n190 = Or(x=w311, y=w308) -> (x .or. y?=w310:bool)
            n191 = In Range and Coerce(upper limit=10.0, x=w316, lower limit=0.0) -> (coerced(x)=w313:dbl)  [unwired: 1 out]
            n192 = Build Array(w325, w322, w323, w324, w319, w319, w319, w319) -> (w321:bool[])
            n193 = case shown="True" w310 {
              tunnel: "Laser Controls" -> [_ w339]
              frame False {
              }
              frame True {
                n194 = call "FPGA-7842R-Control V1.vi"("Action"=FPGA-7842R-Reference."Laser Control", "Laser Controls"=w339, "Initialize"=TRUE) -> ()  [unwired: 11 in, 2 out]
              }
            }
            n195 = Boolean Array To Number(Boolean array=w321) -> (number=w320:u32)
            n196 = To Unsigned Byte Integer(number=w320) -> (unsigned 8bit integer=w318:u8)
            n197 = call "U8_To_U32.vi"("U8 IN"=w318) -> ("U32 OUT"=w317:u32)  [unwired: 13 in, 1 out]
            n198 = call "Volts to I16.vi"("Voltage (V)"=w313) -> ("I16"=w312:i16)  [unwired: 13 in, 1 out]
            n199 = case shown="False" w308 {
              tunnel: "Laser Controls" -> [w337 _]
              frame False {
                n200 = Unbundle By Name(w337) -> ("650 nm"=w334:bool, "590 nm"=w333:bool, "485 nm"=w332:bool)
                n201 = call "Detectors Crl_AE.vi"("Action"=enum16{"READ", "WRITE"}."READ") -> ("Detectors Parameters Out"=w335:T14)  [unwired: 10 in]
                n202 = Bundle By Name(cluster=w335, "Far Red (685/40 nm)"=w334, "Orange (624/40 nm)"=w333, "Green (525/50 nm)"=w332) -> (w331:T14)
                n203 = call "Detectors Crl_AE.vi"("Action"=enum16{"READ", "WRITE"}."WRITE", "Detectors Parameters In"=w331) -> ()  [unwired: 9 in, 1 out]
              }
              frame True {
              }
            }
            n204 = call "Scan Parameters Action Engine.vi"("Action"=enum16{"Read", "Write"}."Read") -> ("Scan Parameters OUT"=w328:T17)  [unwired: 14 in]
            n205 = Bundle By Name(cluster=w328, "Laser_States _U32"=w317, "775_AOM_Volt_I16"=w312) -> (w326:T17)
            n206 = call "Scan Parameters Action Engine.vi"("Action"=enum16{"Read", "Write"}."Write", "Scan Parameters IN"=w326) -> ()  [unwired: 13 in, 1 out]
          }
          frame "Shutters" {
            n207 = Unbundle By Name("Shutters") -> ("Upper Shutter"=w351:bool, "Lower Shutter"=w350:bool)
            n208 = Not(x=w351) -> (.not. x?=w342:bool)
            n209 = Not(x=w350) -> (.not. x?=w341:bool)
            n210 = call "Manual Controls Action Engine.vi"("Action"=enum16{"Read", "Write"}."Read") -> ("Manual Controls Out"=w346:T18)  [unwired: 14 in]
            n211 = Bundle By Name(cluster=w346, "Upper Shutter"=w342, "Lower Shutter"=w341) -> (w343:T18)
            n212 = call "Manual Controls Action Engine.vi"("Action"=enum16{"Read", "Write"}."Write", "Manual Controls In"=w343) -> ()  [unwired: 13 in, 1 out]
            n213 = call "FPGA-7842R-Control V1.vi"("Action"=FPGA-7842R-Reference."Shutter Control", "Manual Controls"=w343, "Initialize"=TRUE) -> ()  [unwired: 11 in, 2 out]
          }
        }
      }
      event Value Change {
        # "For P541 - Sample Z - Converting from Step in µm to I16 is as follows. We have (Step µw)*(10 V / 100 µm)*(32768 I16 / 10 V) = (Step µm)*(32768 I16 / 100 µm) = (Step µm)*(327.68 I16/µm)"
        n214 = event-data() -> ("CtlRef"=w365:refnum<vi>, "OldVal"=w363:variant, "NewVal"=w364:variant)  [unwired: 1 in]
        n215 = local write "Abort AllStage"(FALSE ("Abort AllStage")) -> ()
        n216 = property class="Clust"(reference=w365) -> ("Label.Text"=w362:string)  [unwired: 1 in, 2 out]
        n217 = case shown="\"Sample Z - P541\"" w362 {
          tunnel: w364 -> [_ w388 w429 w456 w519 w560 w589 w628]
          tunnel: w363 -> [_ w387 w428 w455 w520 w561 w590 w629]
          tunnel: ["" "N664" "ASI" "P612" "P612" "P841" "M227" "M686"] -> w361
          tunnel: [dbl[] [0.0] w379 w421 w444 dbl[] [0.0] w549 w582 w618] -> w360
          tunnel: [bool[] [FALSE] w377 w415 w445 bool[] [FALSE] bool[] [TRUE] w583 w617] -> w359
          tunnel: [enum16{"MOVE", "MVR"}."MVR" ("MOVE/MVR") w376 w418 w447 enum16{"MOVE", "MVR"}."MVR" ("MOVE/MVR") w552 w575 w620] -> w358
          tunnel: [0.0 ("Step Size (um)") 0.5 ("Step Size (um)") w420 0.0 ("Velocity") 0.0 ("Velocity") 10000.0 ("Velocity") 0.0 ("Velocity") 0.0 ("Velocity")] -> w354
          tunnel: [StageStates."MVR" ("Action") w374 w419 w448 StageStates."POSITION" ("Action") w553 w579 w621] -> w352
          frame Default {
          }
          frame "Upper Objective Z - N664" {
            n218 = call "N664_Ctrl_Index.vi"("OldVal"=w387, "NewVal"=w388) -> ("Control Ref OUT"=w386:refnum<vi>, "N664 Out"=w384:T5)  [unwired: 12 in]
            n219 = property class="Ctl"(reference=w386) -> ("Label.Text"=w385:string)  [unwired: 1 in, 2 out]
            n220 = Unbundle By Name(w384) -> ("Step Size (um)"=w383:dbl, "Position (mm)"=w382:dbl)
            n221 = case shown="\"Home\"" w385 {
              tunnel: w383 -> [_ w393 w396 _ _ _]
              tunnel: [0.0 ("Step Size (um)") w392 w396 w401 w403 w408] -> w380
              tunnel: w382 -> [_ _ _ w401 w403 _]
              tunnel: [enum16{"MOVE", "MVR"}."MVR" ("MOVE/MVR") enum16{"MOVE", "MVR"}."MVR" ("MOVE/MVR") enum16{"MOVE", "MVR"}."MVR" ("MOVE/MVR") enum16{"MOVE", "MVR"}."MOVE" ("MOVE/MVR") enum16{"MOVE", "MVR"}."MOVE" ("MOVE/MVR") enum16{"MOVE", "MVR"}."MOVE" ("MOVE/MVR")] -> w376
              tunnel: [StageStates."MVR" ("Action") StageStates."MVR" ("Action") StageStates."MVR" ("Action") StageStates."MOVE" ("Action") StageStates."MOVE" ("Action") StageStates."MOVE" ("Action")] -> w374
              frame Default {
              }
              frame "Up N664" {
                n222 = Negate(x=w393) -> (-x=w392:dbl)
              }
              frame "Down N664" {
              }
              frame "Position (mm)" {
              }
              frame "Save" {
                n223 = Build Array(w403) -> (w402:dbl[])
                n224 = call "Stage_position_ae.vi"("Position In"=w402, "StageID"="N664", "Enum"=enum16{"WRITE", "READ", "HOME", "SAVE HOME"}."SAVE HOME") -> ()  [unwired: 7 in, 2 out]
              }
              frame "Home" {
                n225 = call "Stage_position_ae.vi"("StageID"="N664", "Enum"=enum16{"WRITE", "READ", "HOME", "SAVE HOME"}."HOME") -> ("Position Out"=w410:dbl[])  [unwired: 8 in, 1 out]
                n226 = Index Array(array=w410, index=0) -> (element=w408:dbl)
              }
            }
            n227 = Build Array(w380) -> (w379:dbl[])
            n228 = Build Array(TRUE) -> (w377:bool[])
          }
          frame "Cavity Translation Z - ASI" {
            n229 = call "ASI_Ctrl_Index.vi"("NewVal"=w429, "OldVal"=w428) -> ("ASI out"=w425:T6, "Control Ref OUT"=w427:refnum<vi>)  [unwired: 8 in]
            n230 = property class="Ctl"(reference=w427) -> ("Label.Text"=w426:string)  [unwired: 1 in, 2 out]
            n231 = Unbundle By Name(w425) -> ("Step Size (um)"=w424:dbl, "Z (um)"=w423:dbl, "Velocity"=w420:dbl)
            n232 = case shown="\"Z (um)\"" w426 {
              tunnel: w424 -> [_ w435 w438 _]
              tunnel: w423 -> [_ _ _ w442]
              tunnel: [0.0 ("Z (um)") w435 w439 w442] -> w422
              tunnel: [StageStates."MVR" ("Action") StageStates."MVR" ("Action") StageStates."MVR" ("Action") StageStates."MOVE" ("Action")] -> w419
              tunnel: [enum16{"MOVE", "MVR"}."MVR" ("MOVE/MVR") enum16{"MOVE", "MVR"}."MVR" ("MOVE/MVR") enum16{"MOVE", "MVR"}."MVR" ("MOVE/MVR") enum16{"MOVE", "MVR"}."MOVE" ("MOVE/MVR")] -> w418
              frame Default {
              }
              frame "Up ASI" {
              }
              frame "Down ASI" {
                n233 = Negate(x=w438) -> (-x=w439:dbl)
              }
              frame "Z (um)" {
              }
            }
            n234 = Build Array(w422) -> (w421:dbl[])
            n235 = Build Array(TRUE) -> (w415:bool[])
          }
          frame "Bottom Objective XY - P612" {
            n236 = call "P612_Ctrl_Index.vi"("OldVal"=w455, "NewVal"=w456) -> ("Control out"=w454:refnum<vi>, "P612 out"=w452:T9)  [unwired: 12 in]
            n237 = property class="Ctl"(reference=w454) -> ("Label.Text"=w453:string)  [unwired: 1 in, 2 out]
            n238 = Unbundle By Name(w452) -> ("Step Size (um)"=w451:dbl, "X"=w450:dbl, "Y"=w449:dbl)
            n239 = case shown="\"Up Button\"" w453 {
              tunnel: w451 -> [_ _ w467 w474 w478 w485 _]
              tunnel: w450 -> [_ _ _ _ _ _ w492]
              tunnel: w449 -> [_ _ _ _ _ _ w491]
              tunnel: [StageStates."MVR" ("Action") StageStates."HOME" ("Action") StageStates."MVR" ("Action") StageStates."MVR" ("Action") StageStates."MVR" ("Action") StageStates."MVR" ("Action") StageStates."MOVE" ("Action")] -> w448
              tunnel: [enum16{"MOVE", "MVR"}."MVR" ("MOVE/MVR") enum16{"MOVE", "MVR"}."MVR" ("MOVE/MVR") enum16{"MOVE", "MVR"}."MVR" ("MOVE/MVR") enum16{"MOVE", "MVR"}."MVR" ("MOVE/MVR") enum16{"MOVE", "MVR"}."MVR" ("MOVE/MVR") enum16{"MOVE", "MVR"}."MVR" ("MOVE/MVR") enum16{"MOVE", "MVR"}."MOVE" ("MOVE/MVR")] -> w447
              tunnel: [bool[] [FALSE] bool[] [TRUE, TRUE] bool[] [TRUE, FALSE] bool[] [TRUE, FALSE] bool[] [FALSE, TRUE] bool[] [FALSE, TRUE] bool[] [TRUE, TRUE]] -> w445
              tunnel: [dbl[] [0.0] dbl[] [0.0, 0.0] w466 w473 w480 w487 w493] -> w444
              frame Default {
              }
              frame "Home Button" {
              }
              frame "Up Button" {
                n240 = Build Array(w467, 0.0 ("element")) -> (w466:dbl[])
              }
              frame "Down Button" {
                n241 = Negate(x=w474) -> (-x=w471:dbl)
                n242 = Build Array(w471, 0.0 ("element")) -> (w473:dbl[])
              }
              frame "Left Button" {
                n243 = Build Array(0.0 ("element"), w478) -> (w480:dbl[])
              }
              frame "Right Button" {
                n244 = Negate(x=w485) -> (-x=w484:dbl)
                n245 = Build Array(0.0 ("element"), w484) -> (w487:dbl[])
              }
              frame "X", "Y" {
                n246 = Build Array(w492, w491) -> (w493:dbl[])
              }
            }
          }
          frame "Sample Z - P541" {
            w498 = 327.68 ("y")
            n247 = call "P541_Ctrl_Index.vi"("OldVal"=w520, "NewVal"=w519) -> ("Control out"=w518:refnum<vi>, "P541 Out"=w517:T13)  [unwired: 12 in]
            n248 = Unbundle By Name(w517) -> ("Z Position"=w497:dbl, "Step Size (um)"=w516:dbl)
            n249 = property class="Ctl"(reference=w518) -> ("Label.Text"=w515:string)  [unwired: 1 in, 2 out]
            n250 = call "Manual Controls Action Engine.vi"("Action"=enum16{"Read", "Write"}."Read") -> ("Manual Controls Out"=w506:T18)  [unwired: 14 in]
            n251 = Unbundle By Name(w506) -> ("Z Axis Voltage (I16)"=w509:i16)
            n252 = Multiply(x=w497, y=w498) -> (x*y=w512:dbl)
            n253 = Multiply(x=w516, y=w498) -> (x*y=w514:dbl)
            n254 = Round To Nearest(number=w512) -> (nearest integer value=w501:dbl)
            n255 = Round To Nearest(number=w514) -> (nearest integer value=w500:dbl)
            n256 = To Word Integer(number=w501) -> (16bit integer=w511:i16)
            n257 = To Word Integer(number=w500) -> (16bit integer=w513:i16)
            n258 = case shown="\"Step Up\"" w515 {
              tunnel: w513 -> [_ w527 w531 _ _ _]
              tunnel: w511 -> [_ _ _ w533 _ _]
              tunnel: w509 -> [w526 w529 w532 _ w538 _]
              tunnel: [w526 w528 w530 w533 w538 w544] -> w505
              tunnel: w498 -> [_ _ _ _ _ w543]
              tunnel: w497 -> [_ _ _ _ w537 _]
              frame Default {
              }
              frame "Step Down" {
                n259 = Subtract(x=w529, y=w527) -> (x-y=w528:i16)
              }
              frame "Step Up" {
                n260 = Add(x=w532, y=w531) -> (x+y=w530:i16)
              }
              frame "Z Position" {
              }
              frame "Save" {
                n261 = Build Array(w537) -> (w536:dbl[])
                n262 = call "Stage_position_ae.vi"("Position In"=w536, "StageID"="P541", "Enum"=enum16{"WRITE", "READ", "HOME", "SAVE HOME"}."SAVE HOME") -> ()  [unwired: 7 in, 2 out]
              }
              frame "Home" {
                n263 = call "Stage_position_ae.vi"("StageID"="P541", "Enum"=enum16{"WRITE", "READ", "HOME", "SAVE HOME"}."HOME") -> ("Position Out"=w541:dbl[])  [unwired: 8 in, 1 out]
                n264 = Index Array(array=w541, index=0) -> (element=w539:dbl)
                n265 = Multiply(x=w539, y=w543) -> (x*y=w545:dbl)
                n266 = Round To Nearest(number=w545) -> (nearest integer value=w546:dbl)
                n267 = To Word Integer(number=w546) -> (16bit integer=w544:i16)
              }
            }
            n268 = Bundle By Name(cluster=w506, "Z Axis Voltage (I16)"=w505) -> (w508:T18)
            n269 = call "Manual Controls Action Engine.vi"("Action"=enum16{"Read", "Write"}."Write", "Manual Controls In"=w508) -> ("Manual Controls Out"=w502:T18)  [unwired: 13 in]
            n270 = call "FPGA-7842R-Control V1.vi"("Action"=FPGA-7842R-Reference."Stage Control", "Manual Controls"=w502, "Initialize"=TRUE) -> ()  [unwired: 11 in, 2 out]
          }
          frame "Phase Comp Mirror - P841" {
            n271 = call "P841_Ctrl_Index.vi"("OldVal"=w561, "NewVal"=w560) -> ("Control out"=w558:refnum<vi>, "P841 Out"=w556:T7)  [unwired: 12 in]
            n272 = property class="Ctl"(reference=w558) -> ("Label.Text"=w557:string)  [unwired: 1 in, 2 out]
            n273 = Unbundle By Name(w556) -> ("Position (µm)"=w555:dbl, "Step Size (µm)"=w554:dbl)
            n274 = case shown="\"Down P841\"" w557 {
              tunnel: w555 -> [_ _ _ w574]
              tunnel: w554 -> [_ w567 w571 _]
              tunnel: [0.0 ("Position (µm)") w567 w570 w574] -> w550
              tunnel: [StageStates."MVR" ("Action") StageStates."MVR" ("Action") StageStates."MVR" ("Action") StageStates."MOVE" ("Action")] -> w553
              tunnel: [enum16{"MOVE", "MVR"}."MVR" ("MOVE/MVR") enum16{"MOVE", "MVR"}."MVR" ("MOVE/MVR") enum16{"MOVE", "MVR"}."MVR" ("MOVE/MVR") enum16{"MOVE", "MVR"}."MOVE" ("MOVE/MVR")] -> w552
              frame Default {
              }
              frame "Up P841" {
              }
              frame "Down P841" {
                n275 = Negate(x=w571) -> (-x=w570:dbl)
              }
              frame "Position (µm)" {
              }
            }
            n276 = Build Array(w550) -> (w549:dbl[])
          }
          frame "Sample Z Coarse - M227" {
            n277 = call "M227_Ctrl_Index.vi"("OldVal"=w590, "NewVal"=w589) -> ("Control Ref OUT"=w588:refnum<vi>, "M227 Out"=w586:T11)  [unwired: 12 in]
            n278 = property class="Ctl"(reference=w588) -> ("Label.Text"=w587:string)  [unwired: 1 in, 2 out]
            n279 = Unbundle By Name(w586) -> ("Step Size (mm)"=w585:dbl, "MM 1"=w578:dbl, "MM 2"=w577:dbl, "MM 3"=w576:dbl)
            n280 = case shown="\"MM 1\"" w587 {
              tunnel: w585 -> [_ _ _ _ w609 w614]
              tunnel: [bool[] [FALSE, FALSE, FALSE] bool[] [TRUE, TRUE, TRUE] bool[] [TRUE, TRUE, TRUE] bool[] [TRUE, TRUE, TRUE] bool[] [TRUE, TRUE, TRUE] bool[] [TRUE, TRUE, TRUE]] -> w583
              tunnel: [0.0 ("Step Size (mm)") w596 w600 w604 w609 w613] -> w580
              tunnel: [StageStates."POSITION" ("Action") StageStates."MOVE" ("Action") StageStates."MOVE" ("Action") StageStates."MOVE" ("Action") StageStates."MVR" ("Action") StageStates."MVR" ("Action")] -> w579
              tunnel: w578 -> [_ w596 _ _ _ _]
              tunnel: w577 -> [_ _ w600 _ _ _]
              tunnel: w576 -> [_ _ _ w604 _ _]
              tunnel: [enum16{"MOVE", "MVR"}."MVR" ("MOVE/MVR") enum16{"MOVE", "MVR"}."MOVE" ("MOVE/MVR") enum16{"MOVE", "MVR"}."MOVE" ("MOVE/MVR") enum16{"MOVE", "MVR"}."MOVE" ("MOVE/MVR") enum16{"MOVE", "MVR"}."MVR" ("MOVE/MVR") enum16{"MOVE", "MVR"}."MVR" ("MOVE/MVR")] -> w575
              frame Default {
              }
              frame "MM 1" {
              }
              frame "MM 2" {
              }
              frame "MM 3" {
              }
              frame "Up M227" {
              }
              frame "Down M227" {
                n281 = Negate(x=w614) -> (-x=w613:dbl)
              }
            }
            n282 = Build Array(w580, w580, w580) -> (w582:dbl[])
          }
          frame "Sample Stage XY - M686" {
            n283 = call "M686_Ctrl_Index.vi"("NewVal"=w628, "OldVal"=w629) -> ("M686 - out"=w626:T8, "Control out"=w627:refnum<vi>)  [unwired: 8 in]
            n284 = Unbundle By Name(w626) -> ("Step Size (um)"=w625:dbl, "X"=w624:dbl, "Y"=w623:dbl)
            n285 = property class="Ctl"(reference=w627) -> ("Label.Text"=w616:string)  [unwired: 1 in, 2 out]
            n286 = case shown="\"Left Button\"" w616 {
              tunnel: w625 -> [_ _ w641 w646 w654 w659 _]
              tunnel: w624 -> [_ _ _ _ _ _ w666]
              tunnel: w623 -> [_ _ _ _ _ _ w665]
              tunnel: [StageStates."POSITION" ("Action") StageStates."MOVE" ("Action") StageStates."MVR" ("Action") StageStates."MVR" ("Action") StageStates."MVR" ("Action") StageStates."MVR" ("Action") StageStates."MOVE" ("Action")] -> w621
              tunnel: [enum16{"MOVE", "MVR"}."MVR" ("MOVE/MVR") enum16{"MOVE", "MVR"}."MOVE" ("MOVE/MVR") enum16{"MOVE", "MVR"}."MVR" ("MOVE/MVR") enum16{"MOVE", "MVR"}."MVR" ("MOVE/MVR") enum16{"MOVE", "MVR"}."MVR" ("MOVE/MVR") enum16{"MOVE", "MVR"}."MVR" ("MOVE/MVR") enum16{"MOVE", "MVR"}."MOVE" ("MOVE/MVR")] -> w620
              tunnel: [w631 dbl[] [12.5, 12.5] w639 w647 w655 w661 w667] -> w618
              tunnel: [bool[] [FALSE, FALSE] bool[] [TRUE, TRUE] bool[] [TRUE, TRUE] bool[] [TRUE, TRUE] bool[] [TRUE, TRUE] bool[] [TRUE, TRUE] bool[] [TRUE, TRUE]] -> w617
              frame Default {
                w632 = 0.0 ("Step Size (mm)")
                n287 = Build Array(w632, w632) -> (w631:dbl[])
              }
              frame "Home Button" {
              }
              frame "Right Button" {
                n288 = Build Array(w641, 0.0 ("element")) -> (w639:dbl[])
              }
              frame "Left Button" {
                n289 = Negate(x=w646) -> (-x=w645:dbl)
                n290 = Build Array(w645, 0.0 ("element")) -> (w647:dbl[])
              }
              frame "Up Button" {
                n291 = Negate(x=w654) -> (-x=w653:dbl)
                n292 = Build Array(0.0 ("element"), w653) -> (w655:dbl[])
              }
              frame "Down Button" {
                n293 = Build Array(0.0 ("element"), w659) -> (w661:dbl[])
              }
              frame "X", "Y" {
                n294 = Build Array(w666, w665) -> (w667:dbl[])
              }
            }
          }
        }
        n295 = case shown="Default" w362 {
          frame Default {
          }
          frame "Upper Objective Z - N664" {
            n296 = while {
              i -> [w676]
              stop <- w672 stop-if-true
              n297 = call "Stage_position_ae.vi"("StageID"="N664", "Enum"=enum16{"WRITE", "READ", "HOME", "SAVE HOME"}."READ") -> ("Status Out"=w673:bool, "Position Out"=w683:dbl[])  [unwired: 8 in]
              n298 = Greater?(x=w676, y=200) -> (0:w675:bool)
              n299 = And(x=w673, y=w675) -> (x .and. y?=w672:bool)
              n300 = Wait (ms)(milliseconds to wait=u32 1) -> ()  [unwired: 1 out]
              n301 = Index Array(array=w683, index=0) -> (element=w682:dbl)
              n302 = Select(t=u32 16777215, s=w672, f=u32 6618880) -> (s? t:f=w677:u32)
              n303 = property on="Position (mm)" class="DigNum (strict)"("Value"=w682, "NumText.BG Color"=w677) -> ()  [unwired: 2 in, 2 out]
            }
          }
          frame "Cavity Translation Z - ASI" {
            n304 = while {
              shift-right: [w690] -> _
              shift-left: TRUE ("Status Out") -> [w695]
              stop <- w694 stop-if-true
              n305 = call "Stage_position_ae.vi"("StageID"="ASI", "Enum"=enum16{"WRITE", "READ", "HOME", "SAVE HOME"}."READ") -> ("Status Out"=w690:bool, "Position Out"=w698:dbl[])  [unwired: 8 in]
              n306 = Greater?(x=w690, y=w695) -> (0:w694:bool)
              n307 = Wait (ms)(milliseconds to wait=u32 1) -> ()  [unwired: 1 out]
              n308 = Index Array(array=w698, index=0) -> (element=w688:dbl)
              n309 = Divide(x=w688, y=10.0) -> (x/y=w689:dbl)
              n310 = Select(t=u32 16777215, s=w690, f=u32 6618880) -> (s? t:f=w691:u32)
              n311 = property on="Z (um)" class="DigNum (strict)"("Value"=w689, "NumText.BG Color"=w691) -> ()  [unwired: 2 in, 2 out]
            }
          }
        }
        n312 = control-ref of="Abort AllStage"() -> (w353:refnum<vi>)
        n313 = call "AllStage_Limits_Array.vi"("Step(um)/Position(units)"=w360, "Axis"=w359, "Stage ID"=w361, "MOVE/MVR"=w358) -> ("Positions"=w356:dbl[], "Boolean Array"=w355:bool[], "Stage ID"=w357:string)  [unwired: 4 in, 1 out]
        n314 = call "AE_AllStages_Action V2.vi"("Velocity"=w354, "Abort"=w353, "Positions"=w356, "Axis"=w355, "Stage ID"=w357, "Action"=w352) -> ()  [unwired: 3 in, 3 out]
      }
      event "Stages": Value Change {
        n315 = event-data() -> ("NewVal"=w712:T10)  [unwired: 1 in, 2 out]
        n316 = Unbundle By Name(w712) -> ("M686"=w700:bool, "P841"=w710:bool, "ASI"=w708:bool, "N664"=w706:bool, "P612"=w704:bool, "M227"=w702:bool)
        n317 = call "All_Stages_Aloha.vi"("Aloha"=w700, "Stage ID"="M686") -> ()  [unwired: 9 in, 1 out]
        n318 = call "All_Stages_Aloha.vi"("Aloha"=w710, "Stage ID"="P841") -> ()  [unwired: 9 in, 1 out]
        n319 = call "All_Stages_Aloha.vi"("Aloha"=w708, "Stage ID"="ASI") -> ()  [unwired: 9 in, 1 out]
        n320 = call "All_Stages_Aloha.vi"("Aloha"=w706, "Stage ID"="N664") -> ()  [unwired: 9 in, 1 out]
        n321 = call "All_Stages_Aloha.vi"("Aloha"=w704, "Stage ID"="P612") -> ()  [unwired: 9 in, 1 out]
        n322 = call "All_Stages_Aloha.vi"("Aloha"=w702, "Stage ID"="M227") -> ()  [unwired: 9 in, 1 out]
      }
      event "SLM", "Timing", "DM", "Camera", "Focus Lock": Value Change {
        n323 = event-data() -> ("CtlRef"=w716:refnum<vi>, "NewVal"=w713:bool)  [unwired: 1 in, 1 out]
        n324 = property class="Bool (strict)"(reference=w716) -> ("Label.Text"=w715:string)  [unwired: 1 in, 2 out]
        n325 = case shown="\"Focus Lock\"" w715 {
          tunnel: w713 -> [w717 w731 w745 w759 w772]
          frame "SLM", Default {
            n326 = case shown="True" w717 {
              frame False {
                n327 = To Variant(anything=TRUE) -> (Variant=w723:variant)
                n328 = call "SLM AE.vi"("Action"=enum16{"READ", "WRITE"}."READ") -> ("SLM Ref Out"=w724:refnum<vi>)  [unwired: 10 in]
                n329 = invoke class="VI" method="Ctrl Val.Set"(reference=w724, "Control Name"="Exit", "Value"=w723) -> (reference out=w720:refnum<vi>, error out=w719:errorcluster)  [unwired: 2 in, 3 out]
                n330 = invoke on="Hamamatsu LCOS" class="SubPnl" method="Remove VI"(error in=w719) -> (error out=w718:errorcluster)  [unwired: 2 in, 2 out]
                n331 = Close Reference(reference=w720, error in (no error)=w718) -> ()  [unwired: 1 out]
              }
              frame True {
                n332 = Open VI Reference(vi path=path "C:/Users/ED STED/Documents/Test Control Software/Host VIs/SLM_V2/SLM Control.vi") -> (vi reference=w729:refnum<vi>)  [unwired: 5 in, 1 out]
                n333 = invoke class="VI" method="Run VI"(reference=w729, "Wait until done"=FALSE ("Wait Until Done")) -> (reference out=w726:refnum<vi>)  [unwired: 3 in, 4 out]
                n334 = invoke on="Hamamatsu LCOS" class="SubPanel" method="Insert VI"("VI Ref"=w726) -> ()  [unwired: 3 in, 4 out]
                n335 = call "SLM AE.vi"("Action"=enum16{"READ", "WRITE"}."WRITE", "SLM Ref In"=w726) -> ()  [unwired: 9 in, 1 out]
              }
            }
          }
          frame "DM" {
            n336 = case shown="False" w731 {
              frame False {
                n337 = call "DM_Ref_AE.vi"("Action"=enum16{"READ", "WRITE"}."READ") -> ("DM Ref Out"=w738:refnum<vi>)  [unwired: 10 in]
                n338 = To Variant(anything=TRUE) -> (Variant=w737:variant)
                n339 = invoke class="VI" method="Ctrl Val.Set"(reference=w738, "Control Name"="Exit", "Value"=w737) -> (reference out=w734:refnum<vi>, error out=w733:errorcluster)  [unwired: 2 in, 3 out]
                n340 = invoke on="BM Multi" class="SubPnl" method="Remove VI"(error in=w733) -> (error out=w732:errorcluster)  [unwired: 2 in, 2 out]
                n341 = Close Reference(reference=w734, error in (no error)=w732) -> ()  [unwired: 1 out]
              }
              frame True {
                n342 = Open VI Reference(vi path=path "C:/Users/ED STED/Documents/Test Control Software/Host VIs/DM_Dual_V2/Dual_DM_Control_Main_V4.vi") -> (vi reference=w743:refnum<vi>)  [unwired: 5 in, 1 out]
                n343 = invoke class="VI" method="Run VI"(reference=w743, "Wait until done"=FALSE ("Wait Until Done")) -> (reference out=w740:refnum<vi>)  [unwired: 3 in, 4 out]
                n344 = invoke on="BM Multi" class="SubPanel" method="Insert VI"("VI Ref"=w740) -> ()  [unwired: 3 in, 4 out]
                n345 = call "DM_Ref_AE.vi"("Action"=enum16{"READ", "WRITE"}."WRITE", "DM Ref In"=w740) -> ()  [unwired: 9 in, 1 out]
              }
            }
          }
          frame "Timing" {
            n346 = case shown="True" w745 {
              frame False {
                n347 = To Variant(anything=TRUE) -> (Variant=w750:variant)
                n348 = call "GateDelay AE.vi"("Action"=enum16{"READ", "WRITE"}."READ") -> ("Gate Delay Ref Out"=w751:refnum<vi>)  [unwired: 10 in]
                n349 = invoke class="VI" method="Ctrl Val.Set"(reference=w751, "Control Name"="Exit", "Value"=w750) -> (reference out=w746:refnum<vi>, error out=w747:errorcluster)  [unwired: 2 in, 3 out]
                n350 = invoke on="Timing" class="SubPnl" method="Remove VI"(error in=w747) -> (error out=w753:errorcluster)  [unwired: 2 in, 2 out]
                n351 = Close Reference(reference=w746, error in (no error)=w753) -> ()  [unwired: 1 out]
              }
              frame True {
                n352 = Open VI Reference(vi path=path "C:/Users/ED STED/Documents/Test Control Software/Host VIs/Time Delay/GateDelay_Control_V2.vi") -> (vi reference=w756:refnum<vi>)  [unwired: 5 in, 1 out]
                n353 = invoke class="VI" method="Run VI"(reference=w756, "Wait until done"=FALSE ("Wait Until Done")) -> (reference out=w755:refnum<vi>)  [unwired: 3 in, 4 out]
                n354 = invoke on="Timing" class="SubPanel" method="Insert VI"("VI Ref"=w755) -> ()  [unwired: 3 in, 4 out]
                n355 = call "GateDelay AE.vi"("Action"=enum16{"READ", "WRITE"}."WRITE", "Gate Delay Ref In"=w755) -> ()  [unwired: 9 in, 1 out]
              }
            }
          }
          frame "Camera" {
            n356 = case shown="True" w759 {
              frame False {
                n357 = To Variant(anything=TRUE) -> (Variant=w760:variant)
                n358 = call "Camera_Ref_HX.vi"("Action"=enum16{"READ", "WRITE"}."READ") -> ("Alignment Ref Out"=w764:refnum<vi>)  [unwired: 10 in]
                n359 = invoke class="VI" method="Ctrl Val.Set"(reference=w764, "Control Name"="Exit", "Value"=w760) -> (reference out=w763:refnum<vi>)  [unwired: 2 in, 4 out]
                n360 = invoke on="uc480" class="SubPnl" method="Remove VI"() -> (error out=w765:errorcluster)  [unwired: 3 in, 2 out]
                n361 = Close Reference(reference=w763, error in (no error)=w765) -> ()  [unwired: 1 out]
              }
              frame True {
                n362 = Open VI Reference(vi path=path "C:/Users/ED STED/Documents/Test Control Software/Host VIs/Camera/uEye_Control_V1.vi") -> (vi reference=w769:refnum<vi>)  [unwired: 5 in, 1 out]
                n363 = invoke class="VI" method="Run VI"(reference=w769, "Wait until done"=FALSE ("Wait Until Done")) -> (reference out=w768:refnum<vi>)  [unwired: 3 in, 4 out]
                n364 = invoke on="uc480" class="SubPnl" method="Insert VI"("VI Ref"=w768) -> ()  [unwired: 3 in, 4 out]
                n365 = call "Camera_Ref_HX.vi"("Action"=enum16{"READ", "WRITE"}."WRITE", "Alignment Ref In"=w768) -> ()  [unwired: 9 in, 1 out]
              }
            }
          }
          frame "Focus Lock" {
            n366 = case shown="True" w772 {
              frame False {
                n367 = call "Lock Control AE.vi"("Action"=Standard_Action_for_Focus_Lock."Read") -> ("Lock Control  out"=w775:T33)  [unwired: 1 in]
                n368 = Bundle By Name(cluster=w775, "EXIT"=TRUE) -> (w773:T33)
                n369 = call "FocusLock_Ref_HX.vi"("Action"=enum16{"READ", "WRITE"}."READ") -> ("FocusLock Ref Out"=w781:refnum<vi>)  [unwired: 10 in]
                n370 = To Variant(anything=w773) -> (Variant=w779:variant)
                n371 = invoke class="VI" method="Ctrl Val.Set"(reference=w781, "Control Name"="Lock Control", "Value"=w779) -> (reference out=w780:refnum<vi>, error out=w778:errorcluster)  [unwired: 2 in, 3 out]
                n372 = invoke on="Focus Lock\nFocus Lock Panel" class="SubPnl" method="Remove VI"(error in=w778) -> (error out=w782:errorcluster)  [unwired: 2 in, 2 out]
                n373 = Close Reference(reference=w780, error in (no error)=w782) -> ()  [unwired: 1 out]
              }
              frame True {
                n374 = Open VI Reference(vi path=path "C:/Users/ED STED/Documents/Test Control Software/Host VIs/Focus Lock/FocusLock Control.vi") -> (vi reference=w786:refnum<vi>)  [unwired: 5 in, 1 out]
                n375 = invoke class="VI" method="Run VI"(reference=w786, "Wait until done"=FALSE ("Wait Until Done")) -> (reference out=w785:refnum<vi>)  [unwired: 3 in, 4 out]
                n376 = invoke on="Focus Lock\nFocus Lock Panel" class="SubPnl" method="Insert VI"("VI Ref"=w785) -> ()  [unwired: 3 in, 4 out]
                n377 = call "FocusLock_Ref_HX.vi"("Action"=enum16{"READ", "WRITE"}."WRITE", "FocusLock Ref In"=w785) -> ()  [unwired: 9 in, 1 out]
              }
            }
          }
        }
      }
      event Value Change {
        n378 = event-data() -> ("CtlRef"=w794:refnum<vi>, "OldVal"=w792:variant, "NewVal"=w791:variant)  [unwired: 1 in]
        n379 = property class="Clust"(reference=w794) -> ("Label.Text"=w793:string)  [unwired: 1 in, 2 out]
        n380 = call "Graph Ref AE.vi"("Action"=enum16{"READ", "WRITE"}."READ") -> ("Graph Ref Out"=w789:refnum<vi>[])  [unwired: 10 in]
        n381 = case shown="\"Graph Tools\"" w793 {
          tunnel: w792 -> [_ w801 w857]
          tunnel: w791 -> [_ w802 w856]
          tunnel: w789 -> [_ w796 w849]
          frame Default {
          }
          frame "Display Controls" {
            n382 = call "Display_Controls_Ctrl_Index.vi"("OldVal"=w801, "NewVal"=w802) -> ("Control Ref OUT"=w800:refnum<vi>, "Display Controls Out"=w798:T2)  [unwired: 12 in]
            n383 = property class="Ctl"(reference=w800) -> ("Label.Text"=w799:string)  [unwired: 1 in, 2 out]
            n384 = Unbundle By Name(w798) -> ("Single Screen"=w797:bool)
            n385 = case shown="\"Single Screen\", Default" w799 {
              tunnel: w797 -> [w810 _ _]
              tunnel: w796 -> [_ w835 w842]
              frame "Single Screen", Default {
                n386 = property class="App"() -> ("Disp.AllMonitors"=w809:T34)  [unwired: 2 in, 2 out]
                n387 = Index Array(array=w809, index #1=2 ("index"), index #2=0 ("index")) -> (element #1=w806:T35, element #2=w805:T35)
                n388 = control-ref of="This VI"() -> (w804:refnum<vi>)
                n389 = case shown="False" w810 {
                  tunnel: w806 -> [w814 _]
                  tunnel: w805 -> [w813 w825]
                  tunnel: w804 -> [w812 w823]
                  tunnel: T23 {"Left"=0, "Top"=0, "Right"=0, "Bottom"=0} ("Front Panel Window:Window Bounds") -> [w811 w824]
                  frame False {
                    w819 = i16 0
                    n390 = Unbundle By Name(w813) -> ("Bounds.Left"=w816:i16, "Bounds.Bottom"=w817:i16, "Bounds.Top"=w818:i16)
                    n391 = Unbundle By Name(w814) -> ("Bounds.Right"=w815:i16)
                    n392 = Subtract(x=w815, y=w816) -> (x-y=w820:i16)
                    n393 = Subtract(x=w817, y=w818) -> (x-y=w821:i16)
                    n394 = Bundle By Name(cluster=w811, "Left"=w819, "Top"=w819, "Right"=w820, "Bottom"=w821) -> (w822:T23)
                    n395 = property class="VI"(reference=w812, "Front Panel.WinBounds"=w822) -> ()  [unwired: 1 in, 2 out]
                  }
                  frame True {
                    w828 = i16 0
                    n396 = Unbundle By Name(w825) -> ("Bounds.Right"=w831:i16, "Bounds.Bottom"=w830:i16, "Bounds.Top"=w829:i16)
                    n397 = Subtract(x=w830, y=w829) -> (x-y=w827:i16)
                    n398 = Bundle By Name(cluster=w824, "Left"=w828, "Top"=w828, "Right"=w831, "Bottom"=w827) -> (w826:T23)
                    n399 = property class="VI"(reference=w823, "Front Panel.WinBounds"=w826) -> (reference out=w833:refnum<vi>)  [unwired: 1 in, 1 out]
                    n400 = property class="VI"(reference=w833, "FP.State"=T24."Maximized" ("Front Panel Window:State")) -> ()  [unwired: 1 in, 2 out]
                  }
                }
              }
              frame "Add Display" {
                w836 = u16 0 items=["Read", "Write"] ("Action")
                w840 = u16 1 items=["Read", "Write"] ("Action")
                n401 = property on="Add Display" class="Bool (strict)"("Value"=FALSE) -> ()  [unwired: 2 in, 2 out]
                n402 = call "Arange_Displays_V2.vi"("Action"=w836) -> ("Number of Channels OUT"=w837:i32)  [unwired: 14 in]
                n403 = Increment(x=w837) -> (x+1=w839:i32)
                n404 = call "Arange_Displays_V2.vi"("Display References"=w835, "Action"=w840, "Number of Channels"=w839, "Aspect Ratio (h/w)"=1.0) -> ()  [unwired: 11 in, 1 out]
              }
              frame "Remove Display" {
                w843 = u16 0 items=["Read", "Write"] ("Action")
                w847 = u16 1 items=["Read", "Write"] ("Action")
                n405 = call "Arange_Displays_V2.vi"("Action"=w843) -> ("Number of Channels OUT"=w844:i32)  [unwired: 14 in]
                n406 = Decrement(x=w844) -> (x-1=w846:i32)
                n407 = call "Arange_Displays_V2.vi"("Display References"=w842, "Action"=w847, "Number of Channels"=w846, "Aspect Ratio (h/w)"=1.0) -> ()  [unwired: 11 in, 1 out]
                n408 = property on="Remove Display" class="Bool (strict)"("Value"=FALSE) -> ()  [unwired: 2 in, 2 out]
              }
            }
          }
          frame "Graph Tools" {
            n409 = call "Graph_Controls_Ctrl_Index.vi"("OldVal"=w857, "NewVal"=w856) -> ("Control Ref OUT"=w855:refnum<vi>, "Graph Tools Out"=w854:T3)  [unwired: 12 in]
            n410 = property class="Ctl"(reference=w855) -> (reference out=w851:refnum<vi>, "Label.Text"=w850:string)  [unwired: 1 in, 1 out]
            n411 = Unbundle By Name(w854) -> ("Show Cursor"=w853:bool, "Auto Scale"=w852:bool, "Color Map"=w848:T36)
            n412 = case shown="\"Fit Tool\"" w850 {
              selector: w850 -> [_ _ _ w928 _ _ _ _]
              tunnel: w853 -> [_ w897 _ _ _ _ _ _]
              tunnel: w852 -> [_ _ w917 _ _ _ _ _]
              tunnel: w849 -> [w866 w896 w918 w921 w958 w965 w978 w986]
              tunnel: w851 -> [_ _ _ _ _ _ _ _]
              tunnel: w850 -> [_ _ _ w923 _ _ _ _]
              tunnel: w848 -> [w869 _ _ _ _ _ _ _]
              frame "Apply Color" {
                n413 = control-ref of="This VI"() -> (w868:refnum<vi>)
                n414 = call "GetDisplayClick.vi"("Display REFs In"=w866, "Calling VI REF"=w868) -> ("Display Index"=w867:i32)  [unwired: 13 in]
                n415 = Index Array(array=w866, index=w867) -> (element=w865:refnum<vi>)
                n416 = property class="IntGraph (strict)"(reference=w865) -> (reference out=w861:refnum<vi>, error out=w858:errorcluster, "ZScale.Maximum"=w864:dbl)  [unwired: 1 in]
                n417 = case shown="\"Gray\"" w869 {
                  tunnel: [cluster{dbl, u32}[] [{0.0, 0}, {0.07843137254901933, 131072}, {0.15686274509805287, 196608}, {0.235294117647058, 327680}, {0.3137254901960773, 458752}, {0.39215686274509665, 589824}, {0.47058823529410176, 720896}, {0.5490196078431353, 851971}, {0.6274509803921546, 983043}, {0.705882352941174, 1114115}, {0.7843137254902075, 1245187}, {0.8627450980392268, 1376259}, {0.941176470588232, 1507331}, {1.0196078431372513, 1638403}, {1.0980392156862848, 1769475}, {1.1764705882353041, 1769479}, {1.2549019607843093, 2031623}, {1.3333333333333286, 2162695}, {1.4117647058823621, 2293767}, {1.4901960784313673, 2424839}, {1.5686274509803866, 2555911}, {1.647058823529406, 2686983}, {1.7254901960784395, 2818055}, {1.8039215686274588, 2949127}, {1.882352941176464, 3080203}, {1.9607843137254832, 3211275}, {2.0392156862745168, 3342347}, {2.117647058823522, 3473419}, {2.1960784313725554, 3604491}, {2.2745098039215605, 3735563}, {2.352941176470594, 3866635}, {2.431372549019599, 3867403}, {2.5098039215686327, 4129547}, {2.588235294117638, 4260619}, {2.6666666666666714, 4391691}, {2.7450980392156907, 4522763}, {2.823529411764696, 4653839}, {2.901960784313715, 4784911}, {2.9803921568627487, 4915983}, {3.058823529411768, 5178127}, {3.1372549019607874, 5309199}, {3.2156862745097925, 5440271}, {3.294117647058826, 5571343}, {3.3725490196078454, 5702415}, {3.4509803921568647, 5703439}, {3.52941176470587, 5965583}, {3.6078431372549034, 6096655}, {3.6862745098039227, 6227727}, {3.764705882352942, 6358799}, {3.8431372549019756, 6489871}, {3.9215686274509807, 6620943}, {4.0, 6752015}, {4.078431372549019, 6883087}, {4.1568627450980244, 7015183}, {4.235294117647058, 7146255}, {4.313725490196077, 7277327}, {4.392156862745097, 7408399}, {4.470588235294102, 7539471}, {4.549019607843135, 7670543}, {4.627450980392155, 7801615}, {4.705882352941174, 8063759}, {4.784313725490179, 8194831}, {4.862745098039213, 8326927}, {4.941176470588232, 8457999}, {5.019607843137251, 8589075}, {5.098039215686285, 8720147}, {5.17647058823529, 8851219}, {5.254901960784309, 8982291}, {5.333333333333329, 9113363}, {5.411764705882362, 9114387}, {5.490196078431367, 9376531}, {5.568627450980401, 9507603}, {5.647058823529406, 9638675}, {5.7254901960784395, 9769747}, {5.803921568627445, 9901843}, {5.882352941176478, 10032915}, {5.960784313725483, 10163987}, {6.039215686274517, 10229523}, {6.117647058823522, 10295059}, {6.196078431372555, 10427155}, {6.2745098039215605, 10558227}, {6.352941176470594, 10689299}, {6.431372549019599, 10820371}, {6.509803921568633, 10886931}, {6.588235294117638, 10952467}, {6.666666666666671, 11083539}, {6.745098039215691, 11214611}, {6.82352941176471, 11215635}, {6.901960784313715, 11477779}, {6.980392156862749, 11543315}, {7.058823529411768, 11608851}, {7.137254901960787, 11740947}, {7.215686274509821, 11806483}, {7.294117647058826, 11872019}, {7.372549019607845, 12004115}, {7.450980392156865, 12135187}, {7.529411764705898, 12266259}, {7.607843137254903, 12267283}, {7.686274509803923, 12398355}, {7.764705882352942, 12529427}, {7.843137254901947, 12530451}, {7.921568627450981, 12595987}, {8.0, 12530451}, {8.07843137254902, 12793619}, {8.156862745098024, 12794131}, {8.235294117647058, 12794643}, {8.313725490196077, 13056787}, {8.392156862745097, 13057299}, {8.47058823529413, 13057811}, {8.549019607843135, 13188883}, {8.627450980392155, 13320979}, {8.705882352941174, 13386515}, {8.784313725490179, 13452563}, {8.862745098039213, 13584147}, {8.941176470588232, 13584659}, {9.019607843137251, 13585171}, {9.098039215686256, 13585683}, {9.17647058823529, 13717267}, {9.254901960784323, 13848339}, {9.333333333333329, 13849363}, {9.411764705882362, 13849875}, {9.490196078431367, 13850387}, {9.5686274509804, 13981459}, {9.647058823529406, 14113555}, {9.72549019607844, 14114067}, {9.803921568627445, 14114579}, {9.882352941176478, 14115091}, {9.960784313725483, 14246675}, {10.039215686274517, 14377747}, {10.117647058823522, 14378771}, {10.196078431372555, 14379283}, {10.27450980392156, 14379539}, {10.352941176470594, 14379795}, {10.4313725490196, 14380819}, {10.509803921568633, 14511891}, {10.588235294117638, 14643987}, {10.666666666666671, 14644503}, {10.745098039215677, 14645015}, {10.82352941176471, 14645527}, {10.901960784313744, 14646039}, {10.980392156862749, 14646551}, {11.058823529411768, 14778135}, {11.137254901960787, 14909207}, {11.215686274509821, 14910231}, {11.294117647058826, 14910747}, {11.372549019607845, 14911259}, {11.450980392156865, 14911771}, {11.52941176470587, 14912283}, {11.607843137254903, 14912797}, {11.686274509803923, 15044383}, {11.764705882352942, 15175455}, {11.843137254901947, 15175967}, {11.92156862745098, 15176479}, {12.0, 15176991}, {12.07843137254902, 15177507}, {12.156862745098053, 15178019}, {12.235294117647058, 15178531}, {12.313725490196092, 15310115}, {12.392156862745097, 15441701}, {12.47058823529413, 15441959}, {12.549019607843135, 15442215}, {12.627450980392155, 15442727}, {12.705882352941174, 15443243}, {12.784313725490179, 15443755}, {12.862745098039213, 15444269}, {12.941176470588246, 15444783}, {13.019607843137251, 15444783}, {13.098039215686285, 15576367}, {13.17647058823529, 15707953}, {13.25490196078431, 15708467}, {13.333333333333329, 15708979}, {13.411764705882362, 15708981}, {13.490196078431367, 15708983}, {13.568627450980387, 15710011}, {13.647058823529406, 15710523}, {13.725490196078411, 15711037}, {13.803921568627459, 15711039}, {13.882352941176464, 15711553}, {13.960784313725512, 15843139}, {14.039215686274517, 15974213}, {14.117647058823522, 15974215}, {14.196078431372541, 15974217}, {14.27450980392156, 15974219}, {14.352941176470594, 15975755}, {14.431372549019613, 15976271}, {14.509803921568633, 15976785}, {14.588235294117666, 15977299}, {14.666666666666671, 15977301}, {14.745098039215677, 15977815}, {14.82352941176471, 15978327}, {14.901960784313744, 15978331}, {14.980392156862749, 16109917}, {15.058823529411768, 16241503}, {15.137254901960787, 16241505}, {15.215686274509792, 16242019}, {15.294117647058826, 16242535}, {15.372549019607845, 16242537}, {15.450980392156865, 16242539}, {15.529411764705898, 16243563}, {15.607843137254903, 16243567}, {15.686274509803908, 16244081}, {15.764705882352942, 16244595}, {15.843137254901947, 16244599}, {15.92156862745098, 16244601}, {16.0, 16244603}, {16.07843137254902, 16245627}, {16.156862745098024, 16245631}, {16.235294117647058, 16245633}, {16.313725490196077, 16246147}, {16.392156862745097, 16246663}, {16.47058823529413, 16377735}, {16.549019607843135, 16508811}, {16.62745098039217, 16508815}, {16.705882352941174, 16509839}, {16.78431372549018, 16509843}, {16.862745098039213, 16509845}, {16.941176470588232, 16509847}, {17.01960784313725, 16510361}, {17.098039215686256, 16510875}, {17.17647058823529, 16510879}, {17.25490196078431, 16510881}, {17.33333333333333, 16510883}, {17.411764705882362, 16511399}, {17.49019607843138, 16511911}, {17.568627450980387, 16511915}, {17.647058823529406, 16511917}, {17.72549019607844, 16511919}, {17.80392156862746, 16511923}, {17.882352941176464, 16512437}, {17.960784313725483, 16512951}, {18.03921568627449, 16512955}, {18.117647058823522, 16512957}, {18.19607843137254, 16512959}, {18.27450980392156, 16512961}, {18.352941176470594, 16512963}, {18.431372549019613, 16512967}, {18.509803921568633, 16513481}, {18.588235294117638, 16513995}, {18.66666666666667, 16513999}, {18.74509803921569, 16514001}, {18.82352941176471, 16514003}, {18.901960784313744, 16514005}, {18.98039215686275, 16514007}, {19.058823529411754, 16514011}, {19.137254901960787, 16514013}, {19.215686274509792, 16514015}, {19.294117647058826, 16514019}, {19.372549019607845, 16514021}, {19.450980392156865, 16514023}, {19.52941176470587, 16514027}, {19.607843137254918, 16514029}, {19.686274509803923, 16514031}, {19.764705882352942, 16514035}, {19.843137254901947, 16514037}, {19.921568627450995, 16514039}, {20.0, 16514043}] ("Z Scale.Marker Values[]") cluster{dbl, u32}[] [{0.0, 0}, {85.0, 16711680}, {108.0, 16729344}, {127.0, 16744192}, {132.0, 16747520}, {140.0, 16753920}, {157.0, 16766720}, {170.0, 16776960}, {245.0, 16777184}, {250.0, 16777200}, {255.0, 16777215}] ("Z Scale.Marker Values[]") cluster{dbl, u32}[] [{0.0, 0}, {255.0, 16777215}] ("Z Scale.Marker Values[]") cluster{dbl, u32}[] [{0.0, 0}, {255.0, 16711680}] ("Z Scale.Marker Values[]") cluster{dbl, u32}[] [{0.0, 0}, {255.0, 65280}] ("Z Scale.Marker Values[]") cluster{dbl, u32}[] [{0.0, 0}, {255.0, 255}] ("Z Scale.Marker Values[]") cluster{dbl, u32}[] [{0.0, 0}, {255.0, 65535}] ("Z Scale.Marker Values[]") cluster{dbl, u32}[] [{0.0, 0}, {255.0, 16711935}] ("Z Scale.Marker Values[]") cluster{dbl, u32}[] [{0.0, 0}, {255.0, 16776960}] ("Z Scale.Marker Values[]") cluster{dbl, u32}[] [{0.0, 0}, {170.0, 16711680}, {245.0, 16777184}, {250.0, 16777200}, {255.0, 16448250}] ("Z Scale.Marker Values[]") cluster{dbl, u32}[] [{0.0, 0}, {170.0, 65280}, {245.0, 16777184}, {250.0, 16777200}, {255.0, 16448250}] ("Z Scale.Marker Values[]") cluster{dbl, u32}[] [{0.0, 0}, {170.0, 255}, {245.0, 16777184}, {250.0, 16777200}, {255.0, 16448250}] ("Z Scale.Marker Values[]") cluster{dbl, u32}[] [{0.0, 0}, {1.0, 131072}, {2.0, 196608}, {3.0, 327680}, {4.0, 458752}, {5.0, 589824}, {6.0, 720896}, {7.0, 851971}, {8.0, 983043}, {9.0, 1114115}, {10.0, 1245187}, {11.0, 1376259}, {12.0, 1507331}, {13.0, 1638403}, {14.0, 1769475}, {15.0, 1769479}, {16.0, 2031623}, {17.0, 2162695}, {18.0, 2293767}, {19.0, 2424839}, {20.0, 2555911}, {21.0, 2686983}, {22.0, 2818055}, {23.0, 2949127}, {24.0, 3080203}, {25.0, 3211275}, {26.0, 3342347}, {27.0, 3473419}, {28.0, 3604491}, {29.0, 3735563}, {30.0, 3866635}, {31.0, 3867403}, {32.0, 4129547}, {33.0, 4260619}, {34.0, 4391691}, {35.0, 4522763}, {36.0, 4653839}, {37.0, 4784911}, {38.0, 4915983}, {39.0, 5178127}, {40.0, 5309199}, {41.0, 5440271}, {42.0, 5571343}, {43.0, 5702415}, {44.0, 5703439}, {45.0, 5965583}, {46.0, 6096655}, {47.0, 6227727}, {48.0, 6358799}, {49.0, 6489871}, {50.0, 6620943}, {51.0, 6752015}, {52.0, 6883087}, {53.0, 7015183}, {54.0, 7146255}, {55.0, 7277327}, {56.0, 7408399}, {57.0, 7539471}, {58.0, 7670543}, {59.0, 7801615}, {60.0, 8063759}, {61.0, 8194831}, {62.0, 8326927}, {63.0, 8457999}, {64.0, 8589075}, {65.0, 8720147}, {66.0, 8851219}, {67.0, 8982291}, {68.0, 9113363}, {69.0, 9114387}, {70.0, 9376531}, {71.0, 9507603}, {72.0, 9638675}, {73.0, 9769747}, {74.0, 9901843}, {75.0, 10032915}, {76.0, 10163987}, {77.0, 10229523}, {78.0, 10295059}, {79.0, 10427155}, {80.0, 10558227}, {81.0, 10689299}, {82.0, 10820371}, {83.0, 10886931}, {84.0, 10952467}, {85.0, 11083539}, {86.0, 11214611}, {87.0, 11215635}, {88.0, 11477779}, {89.0, 11543315}, {90.0, 11608851}, {91.0, 11740947}, {92.0, 11806483}, {93.0, 11872019}, {94.0, 12004115}, {95.0, 12135187}, {96.0, 12266259}, {97.0, 12267283}, {98.0, 12398355}, {99.0, 12529427}, {100.0, 12530451}, {101.0, 12595987}, {102.0, 12530451}, {103.0, 12793619}, {104.0, 12794131}, {105.0, 12794643}, {106.0, 13056787}, {107.0, 13057299}, {108.0, 13057811}, {109.0, 13188883}, {110.0, 13320979}, {111.0, 13386515}, {112.0, 13452563}, {113.0, 13584147}, {114.0, 13584659}, {115.0, 13585171}, {116.0, 13585683}, {117.0, 13717267}, {118.0, 13848339}, {119.0, 13849363}, {120.0, 13849875}, {121.0, 13850387}, {122.0, 13981459}, {123.0, 14113555}, {124.0, 14114067}, {125.0, 14114579}, {126.0, 14115091}, {127.0, 14246675}, {128.0, 14377747}, {129.0, 14378771}, {130.0, 14379283}, {131.0, 14379539}, {132.0, 14379795}, {133.0, 14380819}, {134.0, 14511891}, {135.0, 14643987}, {136.0, 14644503}, {137.0, 14645015}, {138.0, 14645527}, {139.0, 14646039}, {140.0, 14646551}, {141.0, 14778135}, {142.0, 14909207}, {143.0, 14910231}, {144.0, 14910747}, {145.0, 14911259}, {146.0, 14911771}, {147.0, 14912283}, {148.0, 14912797}, {149.0, 15044383}, {150.0, 15175455}, {151.0, 15175967}, {152.0, 15176479}, {153.0, 15176991}, {154.0, 15177507}, {155.0, 15178019}, {156.0, 15178531}, {157.0, 15310115}, {158.0, 15441701}, {159.0, 15441959}, {160.0, 15442215}, {161.0, 15442727}, {162.0, 15443243}, {163.0, 15443755}, {164.0, 15444269}, {165.0, 15444783}, {166.0, 15444783}, {167.0, 15576367}, {168.0, 15707953}, {169.0, 15708467}, {170.0, 15708979}, {171.0, 15708981}, {172.0, 15708983}, {173.0, 15710011}, {174.0, 15710523}, {175.0, 15711037}, {176.0, 15711039}, {177.0, 15711553}, {178.0, 15843139}, {179.0, 15974213}, {180.0, 15974215}, {181.0, 15974217}, {182.0, 15974219}, {183.0, 15975755}, {184.0, 15976271}, {185.0, 15976785}, {186.0, 15977299}, {187.0, 15977301}, {188.0, 15977815}, {189.0, 15978327}, {190.0, 15978331}, {191.0, 16109917}, {192.0, 16241503}, {193.0, 16241505}, {194.0, 16242019}, {195.0, 16242535}, {196.0, 16242537}, {197.0, 16242539}, {198.0, 16243563}, {199.0, 16243567}, {200.0, 16244081}, {201.0, 16244595}, {202.0, 16244599}, {203.0, 16244601}, {204.0, 16244603}, {205.0, 16245627}, {206.0, 16245631}, {207.0, 16245633}, {208.0, 16246147}, {209.0, 16246663}, {210.0, 16377735}, {211.0, 16508811}, {212.0, 16508815}, {213.0, 16509839}, {214.0, 16509843}, {215.0, 16509845}, {216.0, 16509847}, {217.0, 16510361}, {218.0, 16510875}, {219.0, 16510879}, {220.0, 16510881}, {221.0, 16510883}, {222.0, 16511399}, {223.0, 16511911}, {224.0, 16511915}, {225.0, 16511917}, {226.0, 16511919}, {227.0, 16511923}, {228.0, 16512437}, {229.0, 16512951}, {230.0, 16512955}, {231.0, 16512957}, {232.0, 16512959}, {233.0, 16512961}, {234.0, 16512963}, {235.0, 16512967}, {236.0, 16513481}, {237.0, 16513995}, {238.0, 16513999}, {239.0, 16514001}, {240.0, 16514003}, {241.0, 16514005}, {242.0, 16514007}, {243.0, 16514011}, {244.0, 16514013}, {245.0, 16514015}, {246.0, 16514019}, {247.0, 16514021}, {248.0, 16514023}, {249.0, 16514027}, {250.0, 16514029}, {251.0, 16514031}, {252.0, 16514035}, {253.0, 16514037}, {254.0, 16514039}, {255.0, 16514043}] ("Z Scale.Marker Values[]")] -> w860
                  tunnel: w864 -> [w871 w872 w874 w876 w878 w880 w882 w884 w886 w888 w890 w892 w895]
                  tunnel: [w871 w872 w874 w876 w878 w880 w882 w884 w886 w888 w890 w892 w895] -> w862
                  frame "System", Default {
                  }
                  frame "Fire" {
                    # "Fire"
                  }
                  frame "Gray" {
                    # "Grayscale"
                  }
                  frame "Red" {
                    # "Red"
                  }
                  frame "Green" {
                    # "Green"
                  }
                  frame "Blue" {
                    # "Blue"
                  }
                  frame "Cyan" {
                    # "Cyan"
                  }
                  frame "Magenta" {
                    # "Magenta"
                  }
                  frame "Yellow" {
                    # "Yellow"
                  }
                  frame "Red-White" {
                    # "Red-White"
                  }
                  frame "Green-White" {
                    # "Green-White"
                  }
                  frame "Blue-White" {
                    # "Blue-White"
                  }
                  frame "Glow" {
                  }
                }
                n418 = property on="Apply Color" class="Bool (strict)"(error in=w858, "Value"=FALSE) -> ()  [unwired: 1 in, 2 out]
                n419 = property class="IntGraph (strict)"(reference=w861, "ZScale.MarkerVals[]"=w860, "ZScale.High Color"=u32 255, "ZScale.Maximum"=w862) -> ()  [unwired: 1 in, 2 out]
              }
              frame "Show Cursor", Default {
                w900 = 2.0 ("y")
                n420 = Index Array(array=w896, index=0) -> (element=w908:refnum<vi>)
                n421 = property class="IntGraph (strict)"(reference=w908) -> ("Value"=w907:sgl[][])  [unwired: 1 in, 2 out]
                n422 = Array Size(array=w907) -> (size(s)=w906:i32[])
                n423 = To Double Precision Float(number=w906) -> (double precision float=w903:dbl[])
                n424 = Index Array(array=w903, index #1=0 ("index"), index #2=1 ("index")) -> (element #1=w902:dbl, element #2=w901:dbl)
                n425 = Divide(x=w902, y=w900) -> (x/y=w899:dbl)
                n426 = Divide(x=w901, y=w900) -> (x/y=w898:dbl)
                n427 = for {
                  tunnel: w896 -> [w910] mode=indexing
                  tunnel: w899 -> [w912]
                  tunnel: w898 -> [w911]
                  tunnel: w897 -> [w913]
                  n428 = property class="IntGraph (strict)"(reference=w910, "Cursor.Visible"=w913, "Cursor.Cursor X"=w912, "Cursor.Cursor Y"=w911) -> ()  [unwired: 1 in, 2 out]
                }
              }
              frame "Auto Scale" {
                n429 = Select(t=u8 2 ("Z Scale.Scale Fit"), s=w917, f=u8 0) -> (s? t:f=w914:u8)
                n430 = for {
                  tunnel: w918 -> [w920] mode=indexing
                  tunnel: w914 -> [w919]
                  n431 = property class="IntGraph (strict)"(reference=w920, "ZScale.ScaleFit"=w919) -> ()  [unwired: 1 in, 2 out]
                }
              }
              frame "Pan Tool", "Reset Zoom", "Zoom In", "Zoom Out" {
                n432 = case shown="\"Reset Zoom\"" w928 {
                  tunnel: [0 ("Palette:Active Tool") 6 ("Palette:Active Tool") 7 ("Palette:Active Tool") 1 ("Palette:Active Tool") 0 ("Palette:Active Tool")] -> w922
                  tunnel: w921 -> [_ _ _ _ w940]
                  frame Default {
                  }
                  frame "Zoom In" {
                  }
                  frame "Zoom Out" {
                  }
                  frame "Pan Tool" {
                  }
                  frame "Reset Zoom" {
                    n433 = property on="Reset Zoom" class="Bool (strict)"("Value"=FALSE) -> ()  [unwired: 2 in, 2 out]
                    n434 = for {
                      tunnel: w940 -> [w945] mode=indexing
                      tunnel: 5 ("Palette:Active Tool") -> [w944]
                      n435 = property class="IntGraph (strict)"(reference=w945, "ActPaletteTool"=w944) -> ()  [unwired: 1 in, 2 out]
                    }
                  }
                }
                n436 = control-ref of="Zoom In"() -> (w924:refnum<vi>)
                n437 = control-ref of="Zoom Out"() -> (w926:refnum<vi>)
                n438 = control-ref of="Pan Tool"() -> (w925:refnum<vi>)
                n439 = Build Array(w924, w926, w925) -> (w927:refnum<vi>[])
                n440 = for {
                  tunnel: w927 -> [w933] mode=indexing
                  tunnel: w923 -> [w931]
                  n441 = property class="Bool (strict)"(reference=w933) -> (reference out=w932:refnum<vi>, "Label.Text"=w930:string)  [unwired: 1 in, 1 out]
                  n442 = Equal?(x=w930, y=w931) -> (x = y?=w929:bool)
                  n443 = property class="Bool (strict)"(reference=w932, "Value"=w929) -> ()  [unwired: 1 in, 2 out]
                }
                n444 = for {
                  tunnel: w921 -> [w935] mode=indexing
                  tunnel: w922 -> [w934]
                  n445 = property class="IntGraph (strict)"(reference=w935, "ActPaletteTool"=w934) -> ()  [unwired: 1 in, 2 out]
                }
              }
              frame "Load File" {
                w955 = u16 1 items=["Get Image", "Load and Read File"] ("Action")
                n446 = control-ref of="This VI"() -> (w957:refnum<vi>)
                n447 = property on="Load File" class="Bool (strict)"("Value"=FALSE) -> ()  [unwired: 2 in, 2 out]
                n448 = call "GetDisplayClick.vi"("Display REFs In"=w958, "Calling VI REF"=w957) -> ("Display Index"=w946:i32)  [unwired: 13 in]
                n449 = call "OpenDBL.vi"("Action"=w955) -> ("Image"=w954:sgl[], "Dimensions (Z, Y, X, t)"=w953:i32[])  [unwired: 11 in, 2 out]
                n450 = Index Array(array=w953, index #1=1 ("index"), index #2=2 ("index")) -> (element #1=w950:i32, element #2=w949:i32)
                n451 = Reverse 1D Array(array=w954) -> (reversed array=w948:sgl[])
                n452 = Reshape Array(w948, w950, w949) -> (w947:sgl[][])
                n453 = Index Array(array=w958, index=w946) -> (element=w956:refnum<vi>)
                n454 = property class="IntGraph (strict)"(reference=w956, "Value"=w947) -> ()  [unwired: 1 in, 2 out]
              }
              frame "Fit Tool" {
                n455 = control-ref of="This VI"() -> (w967:refnum<vi>)
                n456 = call "Image Aquisition Param Ctrl_AE.vi"("Action"=enum16{"READ", "WRITE"}."READ") -> ("Image Acquisition Parameters Out"=w962:T16)  [unwired: 10 in]
                n457 = call "GetDisplayClick.vi"("Display REFs In"=w965, "Calling VI REF"=w967) -> ("Display Index"=w966:i32)  [unwired: 13 in]
                n458 = Index Array(array=w965, index=w966) -> (element=w964:refnum<vi>)
                n459 = property class="IntGraph (strict)"(reference=w964) -> ("Value"=w963:sgl[][])  [unwired: 1 in, 2 out]
                n460 = vi-ref "QuickProfile_V3.vi"() -> (w970:refnum<vi>)
                n461 = property class="VI Interface Type 0"(reference=w970) -> ("Path"=w973:path)  [unwired: 1 in, 2 out]
                n462 = Unbundle By Name(w962) -> ("Pixel Size (nm)"=w969:dbl[])
                n463 = Index Array(array=w969, index=0) -> (element=w976:dbl)
                n464 = Open VI Reference(type specifier VI Refnum (for type only)=w970, vi path=w973, options=128) -> (vi reference=w971:refnum<vi>)  [unwired: 3 in, 1 out]
                n465 = call-by-ref "Start Asynchronous Call"(reference=w971, "Image IN"=w963, "Pixel Size (nm)"=w976) -> (reference out=w974:refnum<vi>, error out=w961:errorcluster)  [unwired: 15 in]
                n466 = Close Reference(reference=w974) -> ()  [unwired: 1 in, 1 out]
                n467 = property on="Fit Tool" class="Bool (strict)"(error in=w961, "Value"=FALSE) -> ()  [unwired: 1 in, 2 out]
              }
              frame "Smooth Tool" {
                n468 = vi-ref "SmoothTool.vi"() -> (w981:refnum<vi>)
                n469 = property on="Smooth Tool" class="Bool (strict)"("Value"=FALSE) -> ()  [unwired: 2 in, 2 out]
                n470 = property class="VI Interface Type 1"(reference=w981) -> ("Path"=w983:path)  [unwired: 1 in, 2 out]
                n471 = control-ref of="This VI"() -> (w979:refnum<vi>)
                n472 = Open VI Reference(type specifier VI Refnum (for type only)=w981, vi path=w983, options=128) -> (vi reference=w982:refnum<vi>)  [unwired: 3 in, 1 out]
                n473 = call-by-ref "Start Asynchronous Call"(reference=w982, "Calling VI REF"=w979, "Display REFs In"=w978) -> (reference out=w980:refnum<vi>)  [unwired: 11 in, 1 out]
                n474 = Close Reference(reference=w980) -> ()  [unwired: 1 in, 1 out]
              }
              frame "Merge Tool" {
                n475 = vi-ref "MergeTool - Cambridge.vi"() -> (w989:refnum<vi>)
                n476 = property class="VI Interface Type 2"(reference=w989) -> ("Path"=w991:path)  [unwired: 1 in, 2 out]
                n477 = property on="Merge Tool" class="Bool (strict)"("Value"=FALSE) -> ()  [unwired: 2 in, 2 out]
                n478 = control-ref of="This VI"() -> (w987:refnum<vi>)
                n479 = Open VI Reference(type specifier VI Refnum (for type only)=w989, vi path=w991, options=128) -> (vi reference=w990:refnum<vi>)  [unwired: 3 in, 1 out]
                n480 = call-by-ref "Start Asynchronous Call"(reference=w990, "VI Reference"=w987, "Display References"=w986) -> (reference out=w988:refnum<vi>)  [unwired: 11 in, 1 out]
                n481 = Close Reference(reference=w988) -> ()  [unwired: 1 in, 1 out]
              }
            }
          }
        }
      }
      event "Channel 1", "Channel 2", "Channel 3", "Channel 4", "Channel 5", "Channel 6": Mouse Down; "Channel 1", "Channel 2", "Channel 3", "Channel 4", "Channel 5", "Channel 6": Mouse Up {
        n482 = event-data() -> ("Type"=w998:T25, "CtlRef"=w995:refnum<vi>)  [unwired: 1 in, 5 out]
        n483 = Equal?(x=w998, y=lveventtype."Mouse Down" ("Type")) -> (x = y?=w996:bool)
        n484 = call "Graph Ref AE.vi"("Action"=enum16{"READ", "WRITE"}."READ") -> ("Graph Ref Out"=w993:refnum<vi>[])  [unwired: 10 in]
        n485 = case shown="True" w996 {
          tunnel: w995 -> [w1001 w1019]
          tunnel: w993 -> [w1000 w1018]
          frame False {
            n486 = property class="IntGraph (strict)"(reference=w1001) -> (reference out=w1005:refnum<vi>, "ActPaletteTool"=w1002:i32)  [unwired: 1 in, 1 out]
            n487 = Not Equal?(x=w1002, y=0) -> (x != y?=w1004:bool)
            n488 = case shown="False" w1004 {
              tunnel: w1005 -> [w1008 w1014]
              tunnel: w1000 -> [w1007 w1011]
              frame False {
                n489 = property class="IntGraph (strict)"(reference=w1008) -> ("Cursor.Cursor Position"=w1006:T37)  [unwired: 1 in, 2 out]
                n490 = for {
                  tunnel: w1007 -> [w1009] mode=indexing
                  tunnel: w1006 -> [w1010]
                  n491 = property class="IntGraph (strict)"(reference=w1009, "Cursor.Cursor Position"=w1010) -> ()  [unwired: 1 in, 2 out]
                }
              }
              frame True {
                n492 = property class="IntGraph (strict)"(reference=w1014) -> ("XScale.Range"=w1013:T38, "YScale.Range"=w1012:T38)  [unwired: 1 in, 2 out]
                n493 = for {
                  tunnel: w1013 -> [w1017]
                  tunnel: w1012 -> [w1016]
                  tunnel: w1011 -> [w1015] mode=indexing
                  n494 = property class="IntGraph (strict)"(reference=w1015, "XScale.Range"=w1017, "YScale.Range"=w1016) -> ()  [unwired: 1 in, 2 out]
                }
              }
            }
          }
          frame True {
            n495 = for {
              tunnel: w1018 -> [w1024] mode=indexing
              tunnel: w1019 -> [w1025]
              n496 = Equal?(x=w1024, y=w1025) -> (x = y?=w1023:bool)
              n497 = Select(t=T26 {"Left"=2431, "Top"=-324} ("Z Scale.Position"), s=w1023, f=T26 {"Left"=0, "Top"=0}) -> (s? t:f=w1020:T26)
              n498 = property class="IntGraph (strict)"(reference=w1024, "ZScale.Visible"=w1023, "ZScale.Position"=w1020) -> ()  [unwired: 1 in, 2 out]
            }
          }
        }
      }
      event "Exit": Value Change {
        n499 = event-data() -> ("CtlRef"=w1050:refnum<vi>, "NewVal"=w1052:bool)  [unwired: 1 in, 1 out]
        n500 = Release Notifier(notifier=w1045, force destroy? (F)=TRUE) -> ()  [unwired: 1 in, 3 out]
        n501 = property class="Bool"(reference=w1050) -> ("Label.Text"=w1049:string)  [unwired: 1 in, 2 out]
        n502 = call "SLM AE.vi"("Action"=enum16{"READ", "WRITE"}."READ") -> ("SLM Ref Out"=w1043:refnum<vi>)  [unwired: 10 in]
        n503 = call "DM_Ref_AE.vi"("Action"=enum16{"READ", "WRITE"}."READ") -> ("DM Ref Out"=w1041:refnum<vi>)  [unwired: 10 in]
        n504 = call "GateDelay AE.vi"("Action"=enum16{"READ", "WRITE"}."READ") -> ("Gate Delay Ref Out"=w1042:refnum<vi>)  [unwired: 10 in]
        n505 = Enqueue Element(queue=w1051, element=w1049) -> ()  [unwired: 2 in, 3 out]
        n506 = Build Array(w1043, w1041, w1042) -> (w1040:refnum<vi>[])
        n507 = call "Stage_position_ae.vi"("StageID"="N664", "Enum"=enum16{"WRITE", "READ", "HOME", "SAVE HOME"}."HOME") -> ("Position Out"=w1032:dbl[])  [unwired: 8 in, 1 out]
        n508 = call "Stage_position_ae.vi"("StageID"="P541", "Enum"=enum16{"WRITE", "READ", "HOME", "SAVE HOME"}."HOME") -> ("Position Out"=w1036:dbl[])  [unwired: 8 in, 1 out]
        n509 = for {
          tunnel: w1040 -> [w1057] mode=indexing
          n510 = Not A Number/Path/Refnum?(number/path/refnum=w1057) -> (NaN/Path/Refnum?=w1056:bool)
          n511 = case shown="False" w1056 {
            tunnel: w1057 -> [w1058 _]
            frame False {
              n512 = To Variant(anything=TRUE) -> (Variant=w1059:variant)
              n513 = invoke class="VI" method="Ctrl Val.Set"(reference=w1058, "Control Name"="Exit", "Value"=w1059) -> (reference out=w1062:refnum<vi>)  [unwired: 2 in, 4 out]
              n514 = Close Reference(reference=w1062) -> ()  [unwired: 1 in, 1 out]
            }
            frame True {
            }
          }
        }
        n515 = Index Array(array=w1032, index=0) -> (element=w1029:dbl)
        n516 = property on="Stages" class="Clust (strict)"() -> ("Controls[]"=w1039:refnum<vi>[])  [unwired: 2 in, 2 out]
        n517 = Index Array(array=w1036, index=0) -> (element=w1030:dbl)
        n518 = Build Array(w1030, w1029) -> (w1028:dbl[])
        n519 = for {
          tunnel: w1039 -> [w1055] mode=indexing
          n520 = property class="Ctl"(reference=w1055) -> ("Label.Text"=w1054:string)  [unwired: 1 in, 2 out]
          n521 = call "All_Stages_Aloha.vi"("Aloha"=FALSE, "Stage ID"=w1054) -> ()  [unwired: 9 in, 1 out]
        }
        n522 = call-poly <vilib>:"Write To Spreadsheet File.vi"("format (%.3f)"="%.4f", "1D data"=w1028, "file path (dialog if empty)"=path "C:/Users/ED STED/Documents/Test Control Software/Host VIs/Stages/Stage Positions/home position.csv") -> ()  [unwired: 5 in, 1 out]
      }
    }
  }
  n523 = call "Manual Controls Action Engine.vi"("Action"=enum16{"Read", "Write"}."Write", "Manual Controls In"=w27) -> ("Manual Controls Out"=w29:T18)  [unwired: 13 in]
  n524 = call "FPGA-7842R-Control V1.vi"("Action"=FPGA-7842R-Reference."Initialize", "Manual Controls"=w29, "Initialize"=FALSE) -> ("Initalized"=w11:bool)  [unwired: 11 in, 1 out]
  n525 = while {
    shift-right: [w1075] -> _
    shift-left: "Idle" -> [w1076]
    tunnel: w18 -> [w1072]
    shift-right: [w1070] -> _
    shift-left: w11 -> [w1071]
    tunnel: w1 -> [w1065]
    stop <- w1074 stop-if-true
    n526 = call "Manual Controls Action Engine.vi"("Action"=enum16{"Read", "Write"}."Read") -> ("Manual Controls Out"=w1063:T18)  [unwired: 14 in]
    n527 = call "Image Aquisition Param Ctrl_AE.vi"("Action"=enum16{"READ", "WRITE"}."READ") -> ("Image Acquisition Parameters Out"=w1069:T16)  [unwired: 10 in]
    n528 = call "Detectors Crl_AE.vi"("Action"=enum16{"READ", "WRITE"}."READ") -> ("Detectors Parameters Out"=w1067:T14)  [unwired: 10 in]
    n529 = case shown="\"Arange Displays\"" w1076 {
      selector: w1076 -> [_ _ _ w1109 _ _ _ _ _ _]
      tunnel: ["Exit" w1085 "Idle" ("name (unnamed)") "Arange Displays" ("name (unnamed)") "Start FPGA Acquisition" ("name (unnamed)") "Display" ("name (unnamed)") "Close Images" ("name (unnamed)") "Idle" "Stop Waveforms" ("name (unnamed)") "Start Waveforms" ("name (unnamed)")] -> w1075
      tunnel: [TRUE w1087 w1094 w1117 w1134 w1162 w1203 w1236 w1241 w1247] -> w1074
      tunnel: FALSE -> [_ w1087 w1094 w1117 w1134 w1162 w1203 w1236 w1241 w1247]
      tunnel: w1072 -> [_ w1086 _ _ _ _ _ _ _ _]
      tunnel: w1071 -> [w1081 w1084 w1095 w1115 w1131 w1160 w1201 w1234 w1242 w1248]
      tunnel: [w1080 w1084 w1095 w1115 w1131 w1156 w1201 w1233 w1242 w1248] -> w1070
      tunnel: w1069 -> [_ _ _ w1108 _ w1155 _ _ _ w1245]
      tunnel: w1067 -> [_ _ _ w1107 _ _ _ _ _ w1243]
      tunnel: w1065 -> [_ _ _ _ w1125 _ _ _ _ _]
      tunnel: w1063 -> [_ _ _ w1098 _ _ _ _ _ _]
      frame "Exit" {
        n530 = call "Graph Ref AE.vi"("Action"=enum16{"READ", "WRITE"}."READ") -> ("Graph Ref Out"=w1078:refnum<vi>[])  [unwired: 10 in]
        n531 = call "FPGA-7842R-Control V1.vi"("Action"=FPGA-7842R-Reference."Close FPGA", "Initialize"=w1081) -> ("Initalized"=w1080:bool)  [unwired: 12 in, 1 out]
        n532 = Close Reference(reference=w1078) -> ()  [unwired: 1 in, 1 out]
      }
      frame "Idle", Default {
        n533 = Dequeue Element(queue=w1086, timeout in ms (-1)=-1) -> (element=w1085:string)  [unwired: 1 in, 3 out]
      }
      frame "Close Images" {
        w1090 = u16 0 items=["Read", "Write"] ("Mode")
        w1091 = u16 0 items=["Write", "Read"] ("Mode")
        n534 = call "File Action V1.vi"("Mode"=w1090) -> ("Files Open"=w1089:bool)  [unwired: 12 in, 2 out]
        n535 = call "Image_Actions_V1.vi"("Mode"=w1091, "Action"="Trash Images") -> ()  [unwired: 12 in, 2 out]
        n536 = case shown="True" w1089 {
          frame False {
          }
          frame True {
            w1097 = u16 1 items=["Read", "Write"] ("Mode")
            n537 = call "File Action V1.vi"("Action"="Close Files", "Mode"=w1097) -> ()  [unwired: 11 in, 3 out]
          }
        }
      }
      frame "Capture", "Live" {
        w1113 = u16 0 items=["Write", "Read"] ("Mode")
        n538 = Cluster To Array(cluster=w1107) -> (array=w1105:bool[])
        n539 = Index Array(array=w1105, index=4) -> (element=w1102:bool)
        n540 = Boolean To (0,1)(Boolean=w1105) -> (0, 1=w1106:i16[])
        n541 = Add Array Elements(numeric array=w1106) -> (sum=w1103:i16)
        n542 = To Long Integer(number=w1103) -> (32bit integer=w1100:i32)
        n543 = Unbundle By Name(w1108) -> ("Image Format"=w1110:u16)
        n544 = Select(t=1, s=w1102, f=w1100) -> (s? t:f=w1099:i32)
        n545 = case shown="\"Capture\"" w1109 {
          tunnel: w1108 -> [_ w1120]
          tunnel: w1099 -> [_ w1119]
          tunnel: w1098 -> [_ w1118]
          frame Default {
          }
          frame "Capture" {
            w1123 = u16 1 items=["Read", "Write"] ("Mode")
            n546 = call "File Action V1.vi"("Action"="Open Files", "Mode"=w1123, "Image Acquisition Parameters"=w1120, "Manual Controls In"=w1118, "File Path IN"="Save File Path", "Number of Channels"=w1119) -> ("File Path OUT"=w1121:path)  [unwired: 7 in, 2 out]
            n547 = local write "Save File Path"(w1121) -> ()
          }
        }
        n548 = To Long Integer(number=w1110) -> (32bit integer=w1112:i32)
        n549 = Bundle(w1112, w1112) -> (w1111:cluster{i32, i32})  [unwired: 1 in]
        n550 = call "Image_Actions_V1.vi"("Image Size (Pixels)"=w1111, "Mode"=w1113, "Number of Channels"=w1099, "Action"="Create Images") -> ()  [unwired: 10 in, 2 out]
      }
      frame "Arange Displays" {
        w1129 = u16 1 items=["Write", "Read"] ("Mode")
        w1132 = u16 1 items=["Read", "Write"] ("Action")
        n551 = disable-structure shown="Enabled" {
          disable-tunnel: [w1138 w1139] -> w1126
          disable-tunnel: w1125 -> [w1137 w1139]
          frame Disabled {
            n552 = call "Graph Ref AE.vi"("Action"=enum16{"READ", "WRITE"}."READ", "Graph Ref In"=w1137) -> ("Graph Ref Out"=w1138:refnum<vi>[])  [unwired: 9 in]
          }
          frame Enabled {
          }
        }
        n553 = call "Image_Actions_V1.vi"("Mode"=w1129) -> ("Image REFs OUT"=w1130:T39[])  [unwired: 13 in, 1 out]
        n554 = Array Size(array=w1130) -> (size(s)=w1128:i32)
        n555 = call "Arange_Displays_V2.vi"("Display References"=w1126, "Action"=w1132, "Number of Channels"=w1128, "Aspect Ratio (h/w)"=1.0) -> ("Number of Channels OUT"=w1127:i32)  [unwired: 11 in]
        n556 = for {
          N: w1127 -> [_]
          tunnel: w1126 -> [w1140] mode=indexing
          tunnel: [w1143] -> _ mode=indexing
          i -> [w1141]
          n557 = property class="IntGraph (strict)"(reference=w1140) -> ("Label.Text"=w1145:string)  [unwired: 1 in, 2 out]
          n558 = Equal To 0?(x=w1141) -> (x = 0?=w1142:bool)
          n559 = case shown="True" w1142 {
            tunnel: w1140 -> [_ w1146]
            frame False {
            }
            frame True {
              n560 = property class="IntGraph (strict)"(reference=w1146, "ZScale.Visible"=TRUE ("Z Scale.Visible"), "ZScale.Position"=T26 {"Left"=2431, "Top"=-324} ("Z Scale.Position")) -> ()  [unwired: 1 in, 2 out]
            }
          }
          n561 = To Unsigned Word Integer(number=w1141) -> (unsigned 16bit integer=w1144:u16)
          n562 = Bundle("Label.Text"=w1145, w1144) -> (w1143:cluster{"Label.Text":string, u16})  [unwired: 1 in]
        }
      }
      frame "Start Waveforms" {
        n563 = Unbundle By Name("Laser Controls 2") -> ("Laser On Time (Ticks)"=w1150:i8, "Laser Delay (Ticks)"=w1149:i8)
        n564 = call "Initialize Waveforms V4.vi"("Image Acquisition Parameters"=w1155) -> ("Waveform Data to FPGA"=w1161:T40)  [unwired: 14 in]
        n565 = Unbundle By Name(w1155) -> ("Scan Type"=w1154:enum16{"Sample Scanning", "Beam Scanning"})
        n566 = call "FPGA-7842R-Control V1.vi"("Waveform Data"=w1161, "Action"=FPGA-7842R-Reference."Start Waveforms", "Laser On Time (Ticks)"=w1150, "Image Acquisition Parameters"=w1155, "Initialize"=w1160, "Laser Delay (Ticks)"=w1149) -> ("Initalized"=w1157:bool)  [unwired: 8 in, 1 out]
        n567 = Equal?(x=w1154, y=enum16{"Sample Scanning", "Beam Scanning"}."Sample Scanning" ("Scan Type")) -> (x = y?=w1152:bool)
        n568 = case shown="False" w1152 {
          tunnel: w1157 -> [w1163 w1168]
          tunnel: [w1163 w1167] -> w1156
          frame False {
          }
          frame True {
            n569 = call "Scan Parameters Action Engine.vi"("Action"=enum16{"Read", "Write"}."Read") -> ("Scan Parameters OUT"=w1165:T17)  [unwired: 14 in]
            n570 = Unbundle By Name(w1165) -> ("Unused_Axis_I16"=w1164:i16)
            n571 = call "FPGA-7842R-Control V1.vi"("Action"=FPGA-7842R-Reference."Unused Axis I16", "Initialize"=w1168, "Unused Axis Offset (I16)"=w1164) -> ("Initalized"=w1167:bool)  [unwired: 11 in, 1 out]
          }
        }
      }
      frame "Display" {
        w1196 = u16 1 items=["Write", "Read"] ("Mode")
        n572 = call "Image_Actions_V1.vi"("Mode"=w1196) -> ("Image REFs OUT"=w1198:T39[])  [unwired: 13 in, 1 out]
        n573 = Array Size(array=w1198) -> (size(s)=w1194:i32)
        n574 = Decrement(x=w1194) -> (x-1=w1193:i32)
        n575 = for {
          N: 6 -> [_]
          tunnel: w1193 -> [w1231]
          tunnel: [w1229] -> w1197 mode=indexing
          i -> [w1230]
          n576 = Greater Or Equal?(x=w1231, y=w1230) -> (x >= y?=w1229:bool)
        }
        n577 = Obtain Notifier(name (unnamed)="Running", notification data type=FALSE) -> (notifier out=w1170:refnum<notifier>)  [unwired: 2 in, 2 out]
        n578 = Index Array(array=w1197, index #1=1 ("index"), index #2=2 ("index"), index #3=3 ("index"), index #4=4 ("index"), index #5=5 ("index")) -> (element #1=w1182:bool, element #2=w1181:bool, element #3=w1180:bool, element #4=w1179:bool, element #5=w1178:bool)
        n579 = Index Array(array=w1198, index #1=0 ("index"), index #2=1 ("index"), index #3=2 ("index"), index #4=3 ("index"), index #5=4 ("index"), index #6=5 ("index")) -> (element #1=w1177:T39, element #2=w1176:T39, element #3=w1175:T39, element #4=w1174:T39, element #5=w1173:T39, element #6=w1172:T39)
        n580 = while {
          tunnel: w1182 -> [w1218]
          tunnel: w1181 -> [w1217]
          tunnel: w1180 -> [w1213]
          tunnel: w1179 -> [w1210]
          tunnel: w1178 -> [w1209]
          tunnel: w1177 -> [w1216]
          tunnel: w1176 -> [w1215]
          tunnel: w1175 -> [w1214]
          tunnel: w1174 -> [w1212]
          tunnel: w1173 -> [w1208]
          tunnel: w1172 -> [w1211]
          tunnel: w1170 -> [w1205]
          stop <- w1206 stop-if-true
          n581 = Get Notifier Status(notifier=w1205) -> (current notification=w1206:bool)  [unwired: 1 in, 4 out]
          n582 = case shown="True" w1218 {
            tunnel: w1215 -> [_ w1228]
            frame False {
            }
            frame True {
              n583 = call "IMAQ ImageToArray"("Image"=w1228) -> ("Image Pixels (Float)"=→"Channel 2":sgl[][])  [unwired: 3 in, 4 out]
            }
          }
          n584 = case shown="True" w1217 {
            tunnel: w1214 -> [_ w1226]
            frame False {
            }
            frame True {
              n585 = call "IMAQ ImageToArray"("Image"=w1226) -> ("Image Pixels (Float)"=→"Channel 3":sgl[][])  [unwired: 3 in, 4 out]
            }
          }
          n586 = call "IMAQ ImageToArray"("Image"=w1216) -> ("Image Pixels (Float)"=→"Channel 1":sgl[][])  [unwired: 3 in, 4 out]
          n587 = case shown="True" w1213 {
            tunnel: w1212 -> [_ w1224]
            frame False {
            }
            frame True {
              n588 = call "IMAQ ImageToArray"("Image"=w1224) -> ("Image Pixels (Float)"=→"Channel 4":sgl[][])  [unwired: 3 in, 4 out]
            }
          }
          n589 = case shown="False" w1210 {
            tunnel: w1208 -> [_ w1222]
            frame False {
            }
            frame True {
              n590 = call "IMAQ ImageToArray"("Image"=w1222) -> ("Image Pixels (Float)"=→"Channel 5":sgl[][])  [unwired: 3 in, 4 out]
            }
          }
          n591 = case shown="True" w1209 {
            tunnel: w1211 -> [_ w1220]
            frame False {
            }
            frame True {
              n592 = call "IMAQ ImageToArray"("Image"=w1220) -> ("Image Pixels (Float)"=→"Channel 6":sgl[][])  [unwired: 3 in, 4 out]
            }
          }
          n593 = Wait (ms)(milliseconds to wait=u32 100) -> ()  [unwired: 1 out]
        }
      }
      frame "Stop Waveforms" {
        n594 = call "FPGA-7842R-Control V1.vi"("Action"=FPGA-7842R-Reference."Stop Waveforms", "Initialize"=w1234) -> ("Initalized"=w1233:bool)  [unwired: 12 in, 1 out]
      }
      frame "Stop Acquisition" {
        n595 = call "FPGA-7842R-Control V1.vi"("Action"=FPGA-7842R-Reference."Laser Control", "Laser Controls"=T15 {"STED Power (V)"=0.0, "STED"=FALSE, "650 nm"=FALSE, "590 nm"=FALSE, "485 nm"=FALSE, "Manual Control"=FALSE} ("Laser Controls 2"), "Initialize"=TRUE) -> ()  [unwired: 11 in, 2 out]
      }
      frame "Start FPGA Acquisition" {
        n596 = Unbundle By Name(w1245) -> ("Scan Mode"=w1244:enum16{"XY", "XZ", "YZ", "XYZ"})
        n597 = case shown="\"XZ\", Default" w1244 {
          tunnel: w1245 -> [_ w1255]
          tunnel: w1243 -> [_ w1256]
          frame "YZ" {
            n598 = vi-ref "FPGA Sample Scanning V1.vi"() -> (w1251:refnum<vi>)
            n599 = property class="VI Interface Type 3"(reference=w1251) -> ("Path"=w1249:path)  [unwired: 1 in, 2 out]
            n600 = Open VI Reference(type specifier VI Refnum (for type only)=w1251, vi path=w1249, options=128) -> (vi reference=w1252:refnum<vi>)  [unwired: 3 in, 1 out]
            n601 = call-by-ref "Start Asynchronous Call"(reference=w1252) -> (reference out=w1253:refnum<vi>)  [unwired: 4 in, 1 out]
            n602 = Close Reference(reference=w1253) -> ()  [unwired: 1 in, 1 out]
          }
          frame "XZ", Default {
            n603 = vi-ref "FPGA Beam Scanning V1.vi"() -> (w1254:refnum<vi>)
            n604 = property class="VI Interface Type 5"(reference=w1254) -> ("Path"=w1258:path)  [unwired: 1 in, 2 out]
            n605 = Open VI Reference(type specifier VI Refnum (for type only)=w1254, vi path=w1258, options=128) -> (vi reference=w1257:refnum<vi>)  [unwired: 3 in, 1 out]
            n606 = call-by-ref "Start Asynchronous Call"(reference=w1257, "Detectors"=w1256, "Image Acquisition Parameters"=w1255) -> (reference out=w1260:refnum<vi>)  [unwired: 2 in, 1 out]
            n607 = Close Reference(reference=w1260) -> ()  [unwired: 1 in, 1 out]
          }
        }
      }
    }
  }
